vi "v4.vi"() -> ()   [LabVIEW 2015]
uses:
  <vilib>/Utility/miscctls.llb/LVDateTimeRec.ctl
  <vilib>/Analysis/3filter.llb/Filter Passband Type.ctl
  <vilib>/Analysis/8numeric.llb/1D Numeric Integration.vi
  <vilib>/Utility/inputDevices.llb/mouseAcquire.vi
  <vilib>/Utility/cursorutil.llb/Set Cursor (Icon Pict).vi
  <vilib>/Utility/inputDevices.llb/closeMouse.vi
  <vilib>/Utility/cursorutil.llb/Set Cursor (Cursor ID).vi
  <vilib>/Analysis/3filter.llb/Butterworth Filter (DBL).vi
  <vilib>/Utility/file.llb/Write Delimited Spreadsheet (DBL).vi
  <vilib>/Analysis/NI_AALBase.lvlib
  <vilib>/Analysis/NI_AALPro.lvlib
panel:
  out "TM":string
  out "Vertical (cm/px)":dbl
  out "Horizontal (cm/px)":dbl
  out "Alvo_vertical_px":dbl
  out "Alvo_horizontal_px":dbl
  out "Horizontal_atual_px":i32
  out "Vertical_atual_px":i32
  out "cont6":dbl
  out "cont5":dbl
  out "cont4":dbl
  out "cont2":dbl
  out "cont3":dbl
  out "cont1":dbl
  out "codigo":dbl
  out "Area_acel_1_sub":dbl format="%0.4f"
  out "Area_acel_2_sub":dbl format="%0.4f"
  out "Posicao_final_horizontal":dbl
  out "Posicao_final_Vertical":dbl
  out "Posicao_Hori_2_sub":dbl
  out "Posicao_vert_2_sub":dbl
  out "Deslocamento_Horizontal_fill":dbl[](array[numeric])
  out "Deslocamento_Vertical_fill":dbl[](array[numeric])
  out "Deslocamento_tototal_1_sub":dbl[](array[numeric])
  out "Deslocamento_tototal_2_sub":dbl[](array[numeric])
  out "2_sub_mov(s)":dbl
  out "Fim_da_reposta(s)":dbl format="%#.17g"
  out "Inicio_da_reposta(s)":dbl format="%#.17g"
  out "Apresentacao_do_estimulo(s)":dbl format="%#.17g"
  out "Fim_do_warning(s)":dbl format="%#.17g"
  out "Inicio_do_warning(s)":dbl format="%#.17g"
  out "INICIO(s)":dbl format="%#.17g"
  out "Fim_resp_Cluter":T1
  out "Inicio_da_resposta_Cluter":T1
  out "Apresentacao_do_estimulo_Cluter":T1
  out "Fim_do_warning_Cluter":T1
  out "Inicio_do_warning_Cluter":T1
  out "INICIO_Cluter":T1
  out "x/y":dbl
  out "Fim_do_warning":dbl format="%#.10g"
  out "Inicio_do_warning":dbl format="%#.10g"
  out "Posicao_graus_2_sub":dbl
  out "Posicao_cm_2_sub":dbl
  out "ER_no_2_sub":dbl
  out "Posicao_cm_final":dbl
  out "2_sub_mov":dbl format="%#.10g"
  out "Posicao_graus_final":dbl
  out "Graus":dbl[](array[numeric])
  out "n_correcoes":i32
  out "ref_zero_cross":i32[](array[numeric])
  out "Tempo_relativo_pico":dbl
  out "Tempo_para_o_pico":i32
  out "Pico_velocidade":dbl
  out "Fim_resp":dbl format="%#.10g"
  out "Inicio_da_resposta":dbl format="%#.10g"
  out "Vertical_posicao_px":i32[](array[numeric])
  out "Horizontal_posicao_px":i32[](array[numeric])
  out "Jeark":dbl[](array[numeric])
  out "Deslocamento_Horizontal_bruto":dbl[](array[numeric])
  out "Deslocamento_Vertical_bruto":dbl[](array[numeric])
  out "ref_p_inicial_vertical":dbl
  out "posicao_total":dbl[](array[numeric])
  out "INICIO":dbl format="%#.10g"
  out "Apresentacao_do_estimulo":dbl format="%#.10g"
  out "ref_p_inicial_total":dbl
  out "posicao_horizontal":dbl[](array[numeric])
  out "posicao_vertical":dbl[](array[numeric])
  out "Array_x":dbl[](array[numeric])
  out "ref_t_max":dbl
  out "ref_TR":i32
  out "erro radial (cm)":dbl
  out "meta_precisao":dbl
  out "ref_V_alvo":dbl
  out "ref_H_alvo":dbl
  out "ponto_final":dbl
  out "ref_pont":dbl
  out "Deslocamento_Total__bruto":dbl[](array[numeric])
  out "tentativa":i32
  out "referencia de endereco":path
  out "aceleracao":dbl[](array[numeric])
  out "Velocidade":dbl[](array[numeric])
  out "eixo x":dbl[](array[numeric])
  out "Deslocamento_total_filtrado":dbl[](array[numeric])
  out "cursor":picture
  in  "Tab Control":enum32{"Execucao", "Configuração", "Gráficos"}(tab)
  out "tela":picture
  out "ref_p_inicial_horizontal":dbl
  in  "Cor do ponteiro":u32(colorbox)=14421504
  in  "Cor":u32(colorbox)=197379
  in  "Cor":u32(colorbox)
  in  "Tempo do warning estimulo":u32=1000
  in  "Maior":dbl=4000.0
  in  "menor":dbl=2000.0 format="%#_13g"
  in  "Intervalo entre o fim e o inicio da próxima tentativa":u32=4000
  in  "Horizontal (px)":dbl=1366.0
  in  "Horizontal (cm)":dbl=47.2
  in  "Raio":dbl=1.0
  in  "Horizontal":dbl=5.0
  in  "Vertical":dbl=15.0
  in  "Raio":dbl
  in  "Horizontal":dbl
  in  "Vertical":dbl
  in  "Tamanho do ponteiro":dbl=0.2
  in  "Cor":u32(colorbox)
  in  "Raio":dbl
  in  "Horizontal":dbl
  in  "Sincronizar com EEG":bool
  in  "Número de tentativas":i32=10
  in  "Digite aqui o endereço e nome do arquivo":string
  in  "Tempo max  para fechar a tarefa":dbl=1500.0
  in  "Vertical  (cm)":dbl=29.6
  in  "Vertical (px)":dbl=768.0 format="%#_13g"
  in  "Vertical":dbl=20.0 format="%#_13g"
  in  "Horizontal_1":dbl=31.0
  in  "Vertical_1":dbl=15.0
  in  "Raio_1":dbl=0.3
  in  "Horizontal_1":dbl=31.0
  in  "Vertical_1":dbl=15.0 format="%#_13g"
  in  "Cor_1":u32(colorbox)
  in  "Cor_1":u32(colorbox)
  in  "Raio_1":dbl=0.3
  in  "Horizontal_2":dbl
  in  "Vertical_2":dbl
  in  "Raio_2":dbl
  in  "Horizontal_2":dbl
  in  "Vertical_2":dbl=20.0 format="%#_13g"
  in  "Cor_2":u32(colorbox)
  in  "Cor_2":u32(colorbox)
  in  "Raio_2":dbl
  in  "n_tt_1":dbl=10.0
  in  "n_tt_2":dbl
  in  "Horizontal_3":dbl
  in  "Vertical_3":dbl
  in  "Raio_3":dbl
  in  "Horizontal_3":dbl
  in  "Vertical_3":dbl=20.0 format="%#_13g"
  in  "Cor_3":u32(colorbox)
  in  "Cor_3":u32(colorbox)
  in  "Raio_3":dbl
  in  "n_tt_3":dbl
  in  "n_alvos":dbl=1.0
  in  "Horizontal_4":dbl
  in  "Vertical_4":dbl
  in  "Raio_4":dbl
  in  "Horizontal_4":dbl
  in  "Vertical_4":dbl=20.0 format="%#_13g"
  in  "Cor_4":u32(colorbox)
  in  "Cor_4":u32(colorbox)
  in  "Raio_4":dbl
  in  "n_tt_4":dbl
  in  "Raio_5":dbl
  in  "Cor_5":u32(colorbox)
  in  "Cor_5":u32(colorbox)
  in  "Vertical_5":dbl=20.0 format="%#_13g"
  in  "Horizontal_5":dbl
  in  "Raio_5":dbl
  in  "Vertical_5":dbl
  in  "Horizontal_5":dbl
  in  "n_tt_5":dbl
  in  "Raio_6":dbl
  in  "Cor_6":u32(colorbox)
  in  "Cor_6":u32(colorbox)
  in  "Vertical_6":dbl=20.0 format="%#_13g"
  in  "Horizontal_6":dbl
  in  "Raio_6":dbl
  in  "Vertical_6":dbl
  in  "Horizontal_6":dbl
  in  "n_tt_6":dbl
  in  "Tempo max  do tempo de reaçao":dbl=3000.0
  in  "?":path=path "E:/Programas/Apontamento/versao_vertical/cursor_invisivel.cur"
  in  "FB online":bool
  in  "FB terminal":bool=TRUE
  out "Deslocamento":cluster{"X":dbl[], "Y":dbl[]}[](graph) caption="XY Graph"
  out "Velocidade":cluster{"X":dbl[], "Y":dbl[]}[](graph) caption="XY Graph"
  out "Aceleracao":cluster{"X":dbl[], "Y":dbl[]}[](graph) caption="XY Graph"
  out "Jeark":cluster{"X":dbl[], "Y":dbl[]}[](graph) caption="XY Graph"
  out "Tempo de reação":i32
  out "execucao":picture
  out "Tempo de movimento":i32
  out "home":picture
  # "100 h\n500 v"
  # "800 h\n100 v"
  # "Intervalo aleatória entre o prepara e vai"
  # "entre"
  # "Home"
  # "Ponteiro"
  # "Número de alvos"
  # "Digite aqui o endereço do cursor"
  # "Posição do alvo 1 - Preparação"
  # "Posição do alvo 1 - Execução"
  # "Horizontal"
  # "Horizontal"
  # "Raio"
  # "Raio"
  # "Número de tentativas do alvo"
  # "Vertical"
  # "Vertical"
  # "Posição do alvo 2 - Preparação"
  # "Posição do alvo 2 - Execução"
  # "Horizontal"
  # "Horizontal"
  # "Raio"
  # "Raio"
  # "Número de tentativas do alvo"
  # "Vertical"
  # "Desenvolvido por Tércio Apolinário-Souza"
  # "Vertical"
  # "Posição do alvo 3 - Preparação"
  # "Posição do alvo 3 - Execução"
  # "Horizontal"
  # "Horizontal"
  # "Raio"
  # "Raio"
  # "Número de tentativas do alvo"
  # "Vertical"
  # "Vertical"
  # "Posição do alvo 4 - Execução"
  # "Posição do alvo 4 - Preparação"
  # "Horizontal"
  # "Horizontal"
  # "Raio"
  # "Raio"
  # "Número de tentativas do alvo"
  # "Vertical"
  # "Vertical"
  # "Posição do alvo 5 - Preparação"
  # "Posição do alvo 5 - Execução"
  # "Horizontal"
  # "Horizontal"
  # "Raio"
  # "Raio"
  # "Número de tentativas do alvo"
  # "Vertical"
  # "Vertical"
  # "Posição do alvo 6 - Preparação"
  # "Posição do alvo 6 - Execução"
  # "Horizontal"
  # "Horizontal"
  # "Raio"
  # "Raio"
  # "Número de tentativas do alvo"
  # "Vertical"
  # "Vertical"
  # "Linger"
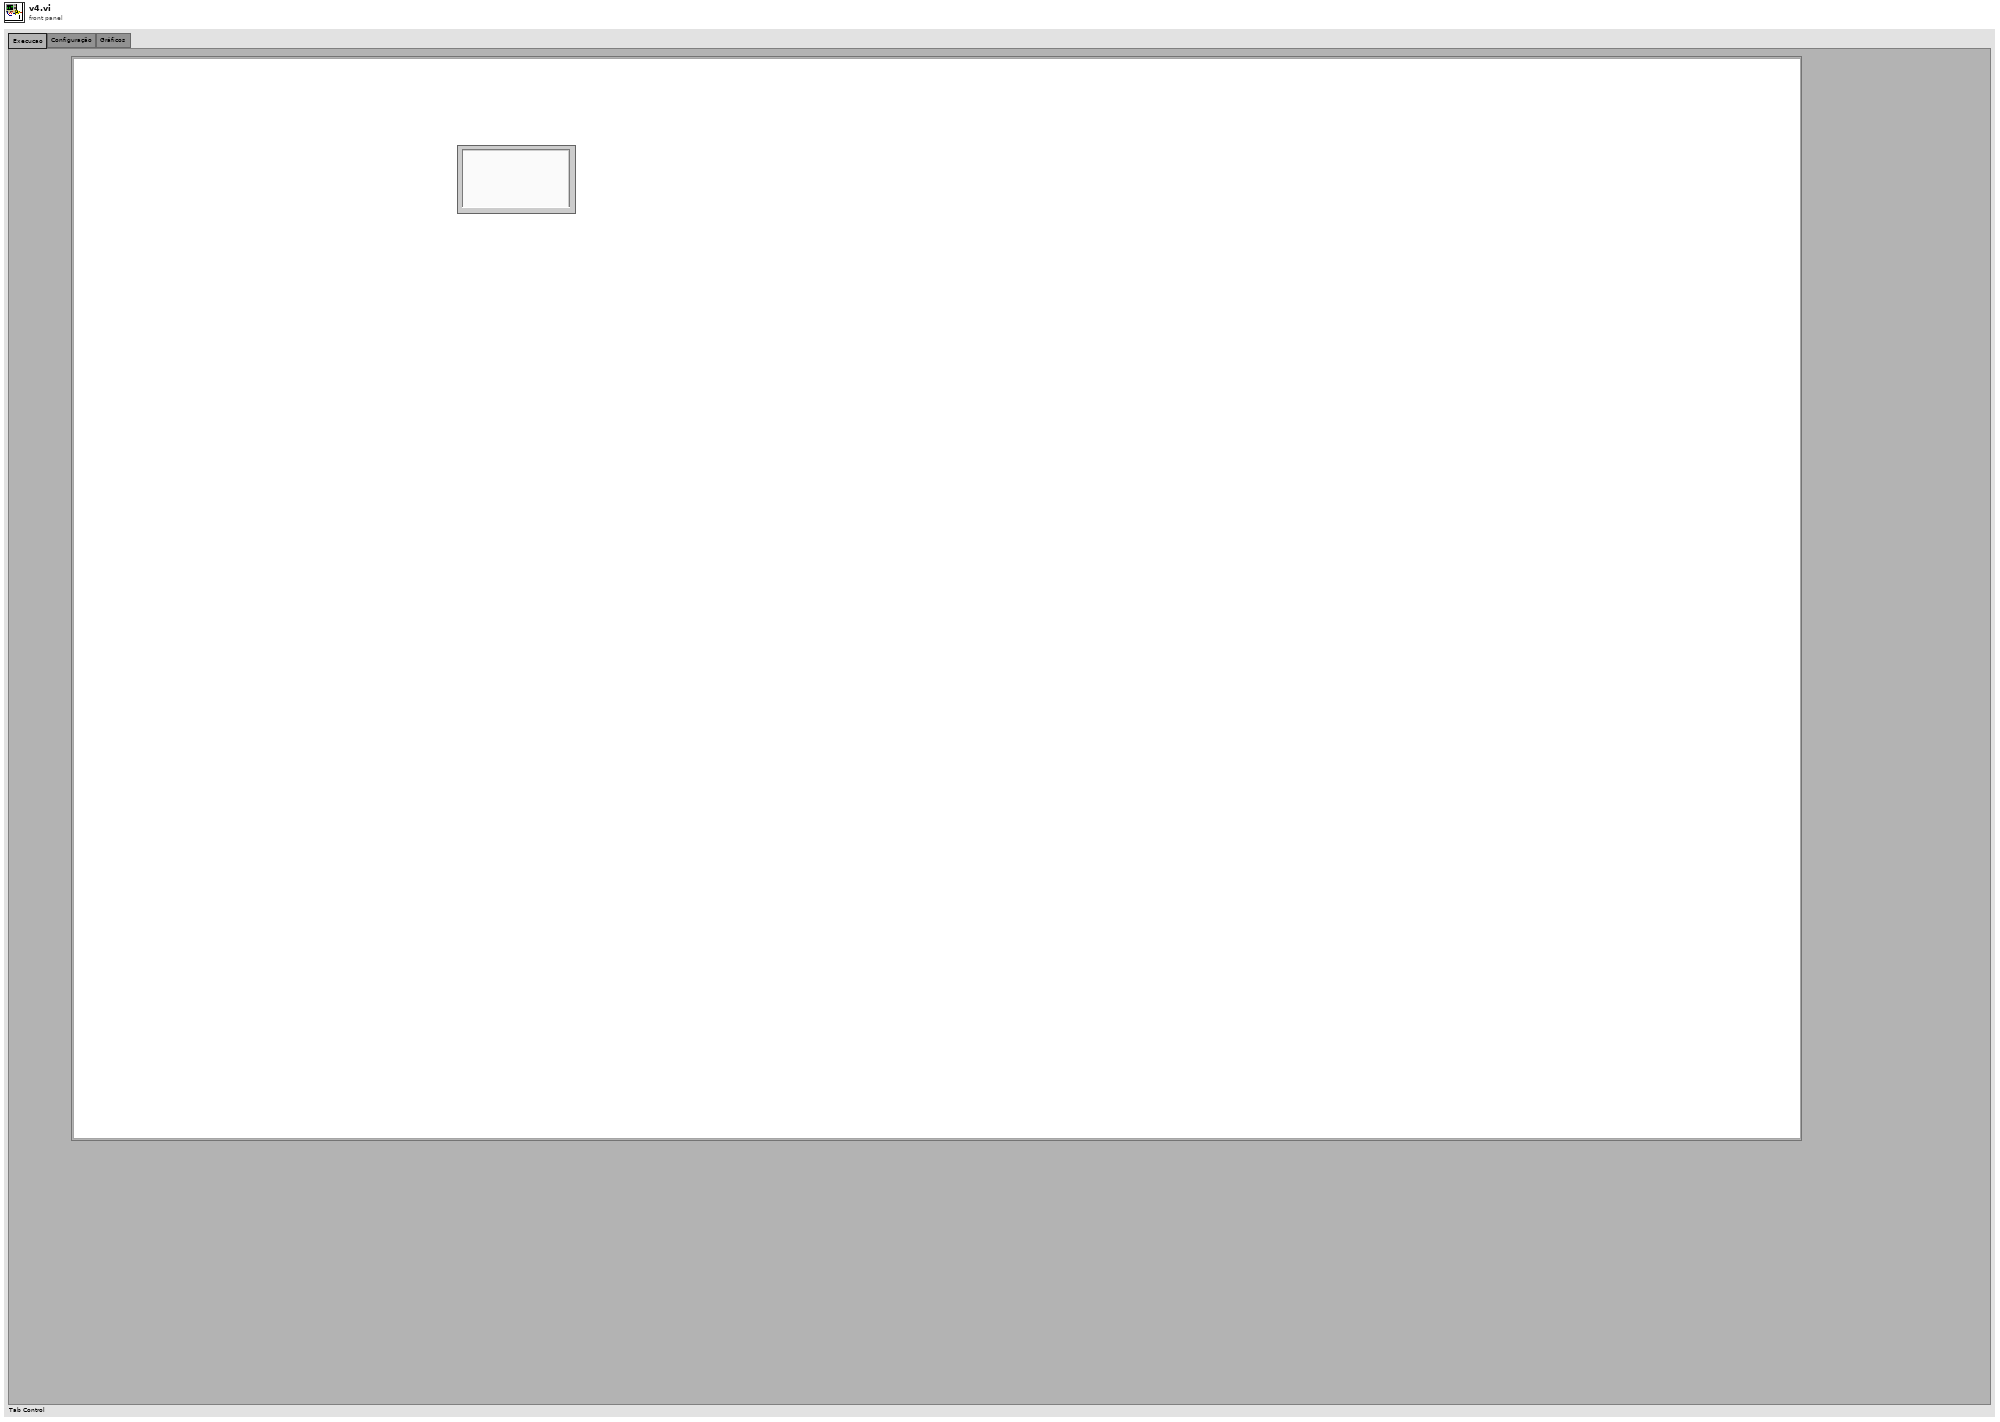
[diagram p1: front panel]
types:
  T1 = typedef "LVDateTimeRec.ctl" = cluster{"fractional second":dbl, "second":i32, "minute":i32, "hour":i32, "day of month":i32, "month":i32, "year":i32, "day of week":i32, "day of year":i32, "DST":i32}
  T2 = typedef "NI_AALBase.lvlib/Filter Passband Type.ctl" = enum32{"Lowpass", "Highpass", "Bandpass", "Bandstop"}
  T3 = cluster{"button 1":bool, "button 2":bool, "button 3":bool, "button 4":bool}
  T4 = cluster{"Horizontal":i32, "Vertical":i32, "Scrolling":i32}
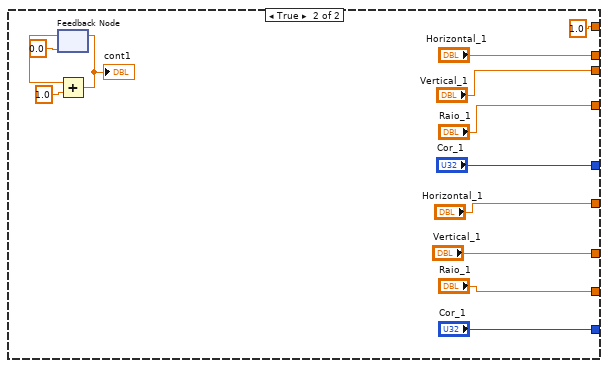
[diagram p4: hidden frame]
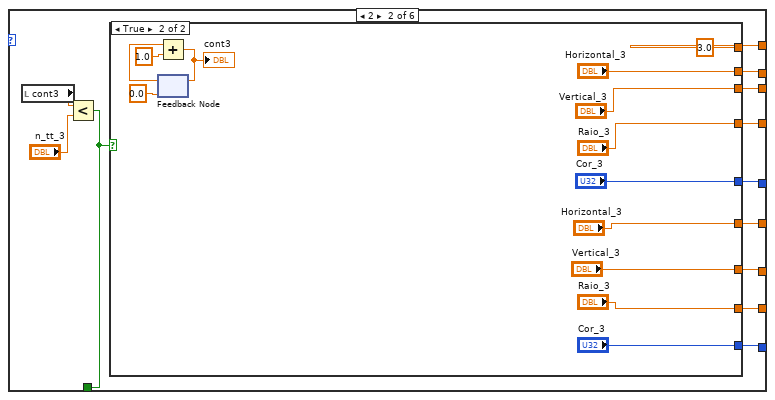
[diagram p5: hidden frame]
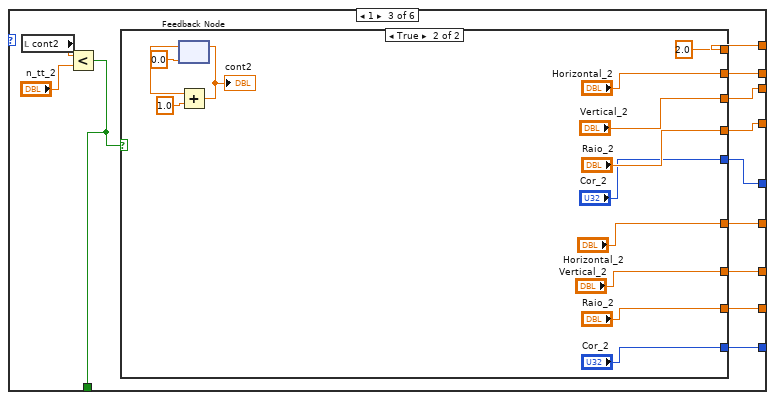
[diagram p7: hidden frame]
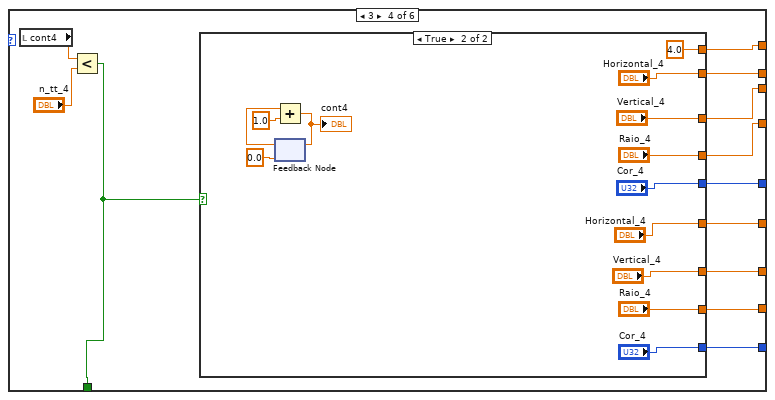
[diagram p9: hidden frame]
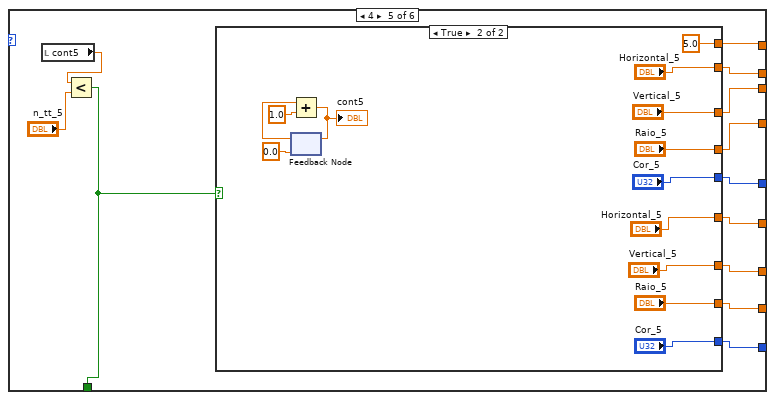
[diagram p11: hidden frame]
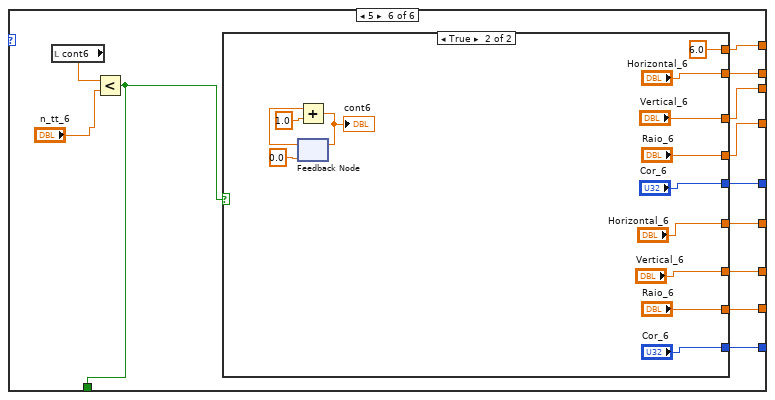
[diagram p13: hidden frame]
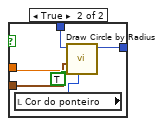
[diagram p20: hidden frame]
diagram:
  w10 = 0.0 ("cont1")
  # "esquerda\ncima\ndireita\nbaixo"
  n1 = local write "cont4"(w10) -> ()
  n2 = local write "cont3"(w10) -> ()
  n3 = local write "cont5"(w10) -> ()
  n4 = local write "cont6"(w10) -> ()
  n5 = local write "cont1"(w10) -> ()
  n6 = local write "cont2"(w10) -> ()
  n7 = for {
    N: "Número de tentativas" -> [_]
    tunnel: [w126] -> w81 mode=indexing
    tunnel: [w125] -> w79 mode=indexing
    tunnel: [w124] -> w77 mode=indexing
    tunnel: [w123] -> w75 mode=indexing
    tunnel: [w122] -> w73 mode=indexing
    tunnel: [w121] -> w71 mode=indexing
    tunnel: [w120] -> w69 mode=indexing
    tunnel: [w119] -> w67 mode=indexing
    tunnel: [w118] -> w65 mode=indexing
    tunnel: [w117] -> w63 mode=indexing
    tunnel: [w116] -> w61 mode=indexing
    tunnel: [w115] -> w59 mode=indexing
    tunnel: [w114] -> w57 mode=indexing
    tunnel: [w113] -> w55 mode=indexing
    tunnel: [w112] -> w52 mode=indexing
    tunnel: [w111] -> w51 mode=indexing
    tunnel: [w110] -> w48 mode=indexing
    tunnel: [w109] -> w47 mode=indexing
    tunnel: [w108] -> w45 mode=indexing
    tunnel: [w107] -> w43 mode=indexing
    tunnel: [w106] -> w41 mode=indexing
    tunnel: [w105] -> w39 mode=indexing
    tunnel: [w104] -> w37 mode=indexing
    tunnel: [w103] -> w35 mode=indexing
    tunnel: [w102] -> w32 mode=indexing
    tunnel: [w101] -> w30 mode=indexing
    tunnel: [w100] -> w29 mode=indexing
    tunnel: [w99] -> w27 mode=indexing
    tunnel: [w98] -> w26 mode=indexing
    tunnel: [w97] -> w24 mode=indexing
    tunnel: [w96] -> w22 mode=indexing
    tunnel: [w95] -> w13 mode=indexing
    tunnel: [w94] -> w19 mode=indexing
    tunnel: [w93] -> w17 mode=indexing
    tunnel: [w92] -> w16 mode=indexing
    tunnel: [w91] -> w9 mode=indexing
    tunnel: [w90] -> w8 mode=indexing
    tunnel: [w89] -> w6 mode=indexing
    tunnel: [w88] -> w4 mode=indexing
    tunnel: [w87] -> w2 mode=indexing
    i -> [w141]
    n8 = Increment(x=w141) -> (x+1=→"tentativa":i32)
    n9 = flat-sequence {
      tunnel: w141 -> [w143]
      tunnel: [w510] -> w139
      tunnel: [w509] -> w134
      tunnel: w139 -> [w608]
      tunnel: [w603] -> w136
      tunnel: [w602] -> w135
      tunnel: w134 -> [w611]
      tunnel: [w601] -> w133
      tunnel: [w696] -> w138
      tunnel: w136 -> [w685]
      tunnel: w135 -> [w679]
      tunnel: w133 -> [w678]
      tunnel: [w676] -> w132
      tunnel: [w677] -> w130
      tunnel: w138 -> [w715]
      tunnel: [w715] -> w137
      tunnel: w132 -> [w702]
      tunnel: [w702] -> w131
      tunnel: w130 -> [w700]
      tunnel: [w700] -> w129
      tunnel: w137 -> [w747]
      tunnel: w131 -> [w744]
      tunnel: w129 -> [w741]
      tunnel: [w880] -> w128
      tunnel: [w880] -> w127
      tunnel: w128 -> [w916]
      tunnel: w127 -> [w928]
      tunnel: [w1125] -> w126
      tunnel: [w1124] -> w125
      tunnel: [w1123] -> w124
      tunnel: [w1122] -> w123
      tunnel: [w1121] -> w122
      tunnel: [w1120] -> w121
      tunnel: [w1119] -> w120
      tunnel: [w1118] -> w119
      tunnel: [w1117] -> w118
      tunnel: [w1116] -> w117
      tunnel: [w1115] -> w116
      tunnel: [w1114] -> w115
      tunnel: [w1113] -> w114
      tunnel: [w1112] -> w113
      tunnel: [w1111] -> w112
      tunnel: [w1110] -> w111
      tunnel: [w1109] -> w110
      tunnel: [w1108] -> w109
      tunnel: [w1107] -> w108
      tunnel: [w1106] -> w107
      tunnel: [w1105] -> w106
      tunnel: [w1104] -> w105
      tunnel: [w1103] -> w104
      tunnel: [w1102] -> w103
      tunnel: [w1101] -> w102
      tunnel: [w1100] -> w101
      tunnel: [w1099] -> w100
      tunnel: [w1098] -> w99
      tunnel: [w1097] -> w98
      tunnel: [w1096] -> w97
      tunnel: [w1095] -> w96
      tunnel: [w1085] -> w95
      tunnel: [w1082] -> w94
      tunnel: [w1094] -> w93
      tunnel: [w1093] -> w92
      tunnel: [w1081] -> w91
      tunnel: [w1080] -> w90
      tunnel: [w1079] -> w89
      tunnel: [w1078] -> w88
      tunnel: [w1077] -> w87
      frame #0 {
        n10 = Equal?(x=w143, y=0) -> (x = y?=w147:bool)
        n11 = And(x="Sincronizar com EEG", y=w147) -> (x .and. y?=w145:bool)
        n12 = case shown="True" w145 {
          frame False {
          }
          frame True {
            n13 = call <vilib>:"Initialize Mouse.vi"() -> ("error out"=w149:errorcluster, "device ID"=w150:refnum<k1>)  [unwired: 10 in]
            n14 = while {
              tunnel: w150 -> [w156]
              tunnel: w149 -> [w155]
              tunnel: enum16{"RELATIVE", "ABSOLUTE"}."ABSOLUTE" ("key mode") -> [w154]
              stop <- w152 stop-if-true
              n15 = call-poly <vilib>:"Acquire Input Data.vi"("device ID"=w156, "key mode"=w154, "error in (no error)"=w155) -> ("button info"=w153:T3)  [unwired: 13 in, 3 out]
              n16 = Unbundle(w153) -> ("button 1"=w151:bool)  [unwired: 3 out]
              n17 = case shown="True" w151 {
                tunnel: [_ TRUE] -> w152
                frame False {
                }
                frame True {
                  n18 = Get Date/Time In Seconds() -> (seconds since 1Jan1904=w158:timestamp)
                  n19 = Format Date/Time String(time format string (%c)="%H%M%S%4u", seconds (now)=w158) -> (date/time string=w160:string)  [unwired: 1 in]
                  n20 = Fract/Exp String To Number(use system decimal point (T)=TRUE, string=w160) -> (number=→"INICIO":dbl)  [unwired: 2 in, 1 out]
                  n21 = Seconds To Date/Time(time stamp (now)=w158) -> (date time rec=→"INICIO_Cluter":T1)  [unwired: 1 in]
                }
              }
            }
          }
        }
        n22 = property on="TM" class="Str"("Visible"=FALSE) -> ()  [unwired: 2 in, 2 out]
      }
      frame #1 {
        n23 = Divide(x="Vertical  (cm)", y="Vertical (px)") -> (x/y=→"Vertical (cm/px)":dbl)
        n24 = Divide(x="Horizontal (cm)", y="Horizontal (px)") -> (x/y=→"Horizontal (cm/px)":dbl)
      }
      frame #2 {
        # "execucao"
        # "Preparacao"
        # "Selecioar alvo"
        n25 = while {
          tunnel: [w188] -> w178
          tunnel: [w187] -> w177
          tunnel: [w186] -> w176
          tunnel: [w185] -> w175
          tunnel: [w184] -> w171
          tunnel: [w183] -> w170
          tunnel: [w182] -> w174
          tunnel: [w181] -> w173
          tunnel: [w179] -> w172
          stop <- w194 stop-if-true
          n26 = Random Number (0-1)() -> (number: 0 to 1=w192:dbl)
          n27 = Multiply(x=w192, y=100.0) -> (x*y=w191:dbl)
          n28 = To Byte Integer(number=w191) -> (8bit integer=w190:i8)
          n29 = Quotient & Remainder(x=w190, y="n_alvos") -> (x-y*floor(x/y)=w189:dbl)  [unwired: 1 out]
          n30 = case shown="0, Default" w189 {
            tunnel: [w206 w231 w256 w278 w306 w327] -> w179
            tunnel: [w204 w229 w254 w280 w296 w329] -> w194
            tunnel: [w203 w228 w253 w277 w305 w328] -> w188
            tunnel: [w202 w227 w252 w276 w304 w326] -> w187
            tunnel: [w201 w226 w251 w275 w303 w325] -> w186
            tunnel: [w200 w225 w250 w274 w302 w324] -> w185
            tunnel: [w199 w224 w249 w273 w301 w323] -> w184
            tunnel: [w198 w223 w248 w272 w300 w322] -> w183
            tunnel: [w197 w222 w247 w271 w299 w321] -> w182
            tunnel: [w196 w221 w246 w270 w298 w320] -> w181
            frame 0, Default {
              n31 = local read "cont1"() -> (w205:dbl)
              n32 = Less?(x=w205, y="n_tt_1") -> (x < y?=w204:bool)
              n33 = case shown="False" w204 {
                tunnel: [_ 1.0] -> w206
                tunnel: [_ "Horizontal_1"] -> w203
                tunnel: [_ "Vertical_1"] -> w202
                tunnel: [_ "Raio_1"] -> w201
                tunnel: [_ "Cor_1"] -> w200
                tunnel: [_ "Horizontal_1"] -> w199
                tunnel: [_ "Vertical_1"] -> w198
                tunnel: [_ "Raio_1"] -> w197
                tunnel: [_ "Cor_1"] -> w196
                frame False {
                }
                frame True {
                  n34 = feedback #1(0.0) -> (w218:dbl)
                  n35 = Add(x=w218, y=1.0) -> (x+y=w215:dbl)
                  "cont1" <- w215
                  n36 = feedback-in #1(w215) -> ()
                }
              }
            }
            frame 2 {
              n37 = local read "cont3"() -> (w230:dbl)
              n38 = Less?(x=w230, y="n_tt_3") -> (x < y?=w229:bool)
              n39 = case shown="True" w229 {
                tunnel: [_ 3.0] -> w231
                tunnel: [_ "Horizontal_3"] -> w228
                tunnel: [_ "Vertical_3"] -> w227
                tunnel: [_ "Raio_3"] -> w226
                tunnel: [_ "Cor_3"] -> w225
                tunnel: [_ "Horizontal_3"] -> w224
                tunnel: [_ "Vertical_3"] -> w223
                tunnel: [_ "Raio_3"] -> w222
                tunnel: [_ "Cor_3"] -> w221
                frame False {
                }
                frame True {
                  n40 = feedback #2(0.0) -> (w242:dbl)
                  n41 = Add(x=w242, y=1.0) -> (x+y=w243:dbl)
                  "cont3" <- w243
                  n42 = feedback-in #2(w243) -> ()
                }
              }
            }
            frame 1 {
              n43 = local read "cont2"() -> (w255:dbl)
              n44 = Less?(x=w255, y="n_tt_2") -> (x < y?=w254:bool)
              n45 = case shown="True" w254 {
                tunnel: [_ 2.0] -> w256
                tunnel: [_ "Horizontal_2"] -> w253
                tunnel: [_ "Vertical_2"] -> w252
                tunnel: [_ "Raio_2"] -> w251
                tunnel: [_ "Cor_2"] -> w250
                tunnel: [_ "Horizontal_2"] -> w249
                tunnel: [_ "Vertical_2"] -> w248
                tunnel: [_ "Raio_2"] -> w247
                tunnel: [_ "Cor_2"] -> w246
                frame False {
                }
                frame True {
                  n46 = feedback #3(0.0) -> (w267:dbl)
                  n47 = Add(x=w267, y=1.0) -> (x+y=w268:dbl)
                  "cont2" <- w268
                  n48 = feedback-in #3(w268) -> ()
                }
              }
            }
            frame 3 {
              n49 = local read "cont4"() -> (w279:dbl)
              n50 = Less?(x=w279, y="n_tt_4") -> (x < y?=w280:bool)
              n51 = case shown="True" w280 {
                tunnel: [_ 4.0] -> w278
                tunnel: [_ "Horizontal_4"] -> w277
                tunnel: [_ "Vertical_4"] -> w276
                tunnel: [_ "Raio_4"] -> w275
                tunnel: [_ "Cor_4"] -> w274
                tunnel: [_ "Horizontal_4"] -> w273
                tunnel: [_ "Vertical_4"] -> w272
                tunnel: [_ "Raio_4"] -> w271
                tunnel: [_ "Cor_4"] -> w270
                frame False {
                }
                frame True {
                  n52 = feedback #4(0.0) -> (w293:dbl)
                  n53 = Add(x=w293, y=1.0) -> (x+y=w294:dbl)
                  "cont4" <- w294
                  n54 = feedback-in #4(w294) -> ()
                }
              }
            }
            frame 4 {
              n55 = local read "cont5"() -> (w295:dbl)
              n56 = Less?(x=w295, y="n_tt_5") -> (x < y?=w296:bool)
              n57 = case shown="True" w296 {
                tunnel: [_ 5.0] -> w306
                tunnel: [_ "Horizontal_5"] -> w305
                tunnel: [_ "Vertical_5"] -> w304
                tunnel: [_ "Raio_5"] -> w303
                tunnel: [_ "Cor_5"] -> w302
                tunnel: [_ "Horizontal_5"] -> w301
                tunnel: [_ "Vertical_5"] -> w300
                tunnel: [_ "Raio_5"] -> w299
                tunnel: [_ "Cor_5"] -> w298
                frame False {
                }
                frame True {
                  n58 = feedback #5(0.0) -> (w318:dbl)
                  n59 = Add(x=w318, y=1.0) -> (x+y=w319:dbl)
                  "cont5" <- w319
                  n60 = feedback-in #5(w319) -> ()
                }
              }
            }
            frame 5 {
              n61 = local read "cont6"() -> (w330:dbl)
              n62 = Less?(x=w330, y="n_tt_6") -> (x < y?=w329:bool)
              n63 = case shown="True" w329 {
                tunnel: [_ 6.0] -> w327
                tunnel: [_ "Horizontal_6"] -> w328
                tunnel: [_ "Vertical_6"] -> w326
                tunnel: [_ "Raio_6"] -> w325
                tunnel: [_ "Cor_6"] -> w324
                tunnel: [_ "Horizontal_6"] -> w323
                tunnel: [_ "Vertical_6"] -> w322
                tunnel: [_ "Raio_6"] -> w321
                tunnel: [_ "Cor_6"] -> w320
                frame False {
                }
                frame True {
                  n64 = feedback #6(0.0) -> (w343:dbl)
                  n65 = Add(x=w343, y=1.0) -> (x+y=w344:dbl)
                  "cont6" <- w344
                  n66 = feedback-in #6(w344) -> ()
                }
              }
            }
          }
        }
        "codigo" <- w172
        n67 = local write "Horizontal"(w178) -> ()
        n68 = local write "Vertical"(w177) -> ()
        n69 = local write "Horizontal"(w171) -> ()
        n70 = local write "Raio"(w174) -> ()
        n71 = local write "Cor"(w175) -> ()
        n72 = local write "Vertical"(w170) -> ()
        n73 = local write "Raio"(w176) -> ()
        n74 = local write "Cor"(w173) -> ()
      }
      frame #3 {
        # "voltar o mouse ao normal"
        # "Preparação"
        n75 = call <vilib>:"Initialize Mouse.vi"() -> ("error out"=w348:errorcluster, "device ID"=w349:refnum<k1>)  [unwired: 10 in]
        n76 = while {
          tunnel: w349 -> [w401]
          tunnel: w348 -> [w394]
          tunnel: [w376] -> w347
          tunnel: [w395] -> w346
          stop <- w396 stop-if-true
          # "Alvo 1"
          n77 = local read "Vertical  (cm)"() -> (w374:dbl)
          n78 = local read "Horizontal (cm/px)"() -> (w353:dbl)
          n79 = call-poly <vilib>:"Acquire Input Data.vi"("device ID"=w401, "error in (no error)"=w394) -> ("device ID"=w376:refnum<k1>, "axis info"=w400:T4, "error out"=w395:errorcluster)  [unwired: 14 in, 1 out]
          n80 = Subtract(x=w374, y="Vertical") -> (x-y=w373:dbl)
          n81 = Divide(x=w373, y=w353) -> (x/y=w352:dbl)
          n82 = Unbundle By Name(w400) -> ("Vertical"=w368:i32, "Horizontal"=w371:i32)
          n83 = Divide(x="Horizontal", y=w353) -> (x/y=w377:dbl)
          n84 = Divide(x="Raio", y=w353) -> (x/y=w360:dbl)
          "x/y" <- w360
          n85 = Bundle(w377, w352) -> (w384:cluster{dbl, dbl})  [unwired: 1 in]
          n86 = Quotient & Remainder(x=w377, y=1.0) -> (floor(x/y)=w370:dbl)  [unwired: 1 out]
          n87 = Quotient & Remainder(x=w352, y=1.0) -> (floor(x/y)=w367:dbl)  [unwired: 1 out]
          n88 = call <vilib>:"Draw Circle by Radius.vi"("color(black)"="Cor", "fill?(F)"=TRUE, "pixel center"=w384, "radius"=w360) -> ("new picture"=w385:picture)  [unwired: 7 in]
          "home" <- w385
          n89 = Subtract(x=w371, y=w370) -> (x-y=w369:dbl)
          n90 = local read "Horizontal (cm/px)"() -> (w386:dbl)
          n91 = Subtract(x=w368, y=w367) -> (x-y=w366:dbl)
          n92 = Absolute Value(x=w369) -> (abs(x)=w363:dbl)
          n93 = local read "Vertical  (cm)"() -> (w375:dbl)
          n94 = local read "Vertical"() -> (w356:dbl)
          n95 = local read "Horizontal (cm/px)"() -> (w381:dbl)
          n96 = local read "Raio"() -> (w357:dbl)
          n97 = local read "Horizontal"() -> (w358:dbl)
          n98 = Absolute Value(x=w366) -> (abs(x)=w362:dbl)
          n99 = Divide(x=w360, y=2.0) -> (x/y=w359:dbl)
          n100 = Less Or Equal?(x=w362, y=w359) -> (x <= y?=w364:bool)
          n101 = Less Or Equal?(x=w363, y=w359) -> (x <= y?=w365:bool)
          n102 = Bundle("Horizontal"=w371, "Vertical"=w368) -> (w399:cluster{"Horizontal":i32, "Vertical":i32})  [unwired: 1 in]
          n103 = Subtract(x=w375, y=w356) -> (x-y=w372:dbl)
          n104 = And(x=w364, y=w365) -> (x .and. y?=w396:bool)
          n105 = Divide(x=w372, y=w386) -> (x/y=w350:dbl)
          "ref_V_alvo" <- w350
          n106 = Divide(x=w357, y=w386) -> (x/y=w390:dbl)
          n107 = Divide(x=w358, y=w386) -> (x/y=w351:dbl)
          "ref_H_alvo" <- w351
          n108 = Divide(x="Tamanho do ponteiro", y=w381) -> (x/y=w380:dbl)
          "ref_pont" <- w380
          n109 = Bundle(w351, w350) -> (w387:cluster{dbl, dbl})  [unwired: 1 in]
          n110 = local read "Cor"() -> (w355:u32)
          n111 = call <vilib>:"Draw Circle by Radius.vi"("color(black)"=w355, "fill?(F)"=TRUE, "pixel center"=w387, "radius"=w390, "picture"=w385) -> ("new picture"=w389:picture)  [unwired: 6 in]
          "cursor" <- w389
          n112 = call <vilib>:"Draw Circle by Radius.vi"("color(black)"="Cor do ponteiro", "fill?(F)"=TRUE, "pixel center"=w399, "radius"=w380, "picture"=w389) -> ("new picture"=→"tela":picture)  [unwired: 6 in]
        }
        n113 = call-poly <vilib>:"Set Cursor.vi"("icon"=i16 0 ("cursor resource ID")) -> ()  [unwired: 9 in, 2 out]
        n114 = call-poly <vilib>:"Close Input Device.vi"("error in (no error)"=w346, "device ID"=w347) -> ()  [unwired: 8 in, 1 out]
      }
      frame #4 {
      }
      frame #5 {
        n115 = case shown="True" TRUE {
          frame False {
          }
          frame True {
            n116 = Get Date/Time In Seconds() -> (seconds since 1Jan1904=w409:timestamp)
            n117 = Format Date/Time String(time format string (%c)="%H%M%S%4u", seconds (now)=w409) -> (date/time string=w411:string)  [unwired: 1 in]
            n118 = Fract/Exp String To Number(use system decimal point (T)=TRUE, string=w411) -> (number=→"Inicio_do_warning":dbl)  [unwired: 2 in, 1 out]
            n119 = Seconds To Date/Time(time stamp (now)=w409) -> (date time rec=→"Inicio_do_warning_Cluter":T1)  [unwired: 1 in]
          }
        }
        n120 = Wait (ms)(milliseconds to wait="Tempo do warning estimulo") -> ()  [unwired: 1 out]
        n121 = call <vilib>:"Beep.vi"("use system alert? (T)"=FALSE, "duration (msec)"=u32 200, "frequency (Hz)"=u32 500) -> ()  [unwired: 9 in]
      }
      frame #6 {
        # "ocultar o mouse"
        # "intervalo entre 1 a 3 segundo"
        # "Isso serve para apagar"
        n122 = case shown="True" TRUE {
          frame False {
          }
          frame True {
            n123 = Get Date/Time In Seconds() -> (seconds since 1Jan1904=w425:timestamp)
            n124 = Format Date/Time String(time format string (%c)="%H%M%S%4u", seconds (now)=w425) -> (date/time string=w428:string)  [unwired: 1 in]
            n125 = Fract/Exp String To Number(use system decimal point (T)=TRUE, string=w428) -> (number=→"Fim_do_warning":dbl)  [unwired: 2 in, 1 out]
            n126 = Seconds To Date/Time(time stamp (now)=w425) -> (date time rec=→"Fim_do_warning_Cluter":T1)  [unwired: 1 in]
          }
        }
        n127 = Random Number (0-1)() -> (number: 0 to 1=w418:dbl)
        n128 = Subtract(x="Maior", y=1.0) -> (x-y=w423:dbl)
        n129 = call <vilib>:"Draw Circle by Radius.vi"() -> ("new picture"=w417:picture)  [unwired: 11 in]
        n130 = Multiply(x=w423, y=w418) -> (x*y=w419:dbl)
        n131 = Add(x=w419, y="menor") -> (x+y=w424:dbl)
        n132 = local write "tela"(w417) -> ()
        n133 = Wait (ms)(milliseconds to wait=w424) -> ()  [unwired: 1 out]
        n134 = call <vilib>:"Create Cursor From File.vi"("cursor file"="?") -> ("cursor ID"=w415:refnum<k1>)  [unwired: 9 in, 1 out]
        n135 = call-poly <vilib>:"Set Cursor.vi"("cursor ID"=w415) -> ()  [unwired: 9 in, 2 out]
      }
      frame #7 {
        w439 = dbl[] [0.0]
        # "Tempo reação"
        n136 = call <vilib>:"Initialize Mouse.vi"() -> ("error out"=w441:errorcluster, "device ID"=w442:refnum<k1>)  [unwired: 10 in]
        n137 = case shown="True" TRUE {
          frame False {
          }
          frame True {
            n138 = Get Date/Time In Seconds() -> (seconds since 1Jan1904=w443:timestamp)
            n139 = Format Date/Time String(time format string (%c)="%H%M%S%4u", seconds (now)=w443) -> (date/time string=w446:string)  [unwired: 1 in]
            n140 = Fract/Exp String To Number(use system decimal point (T)=TRUE, string=w446) -> (number=→"Apresentacao_do_estimulo":dbl)  [unwired: 2 in, 1 out]
            n141 = Seconds To Date/Time(time stamp (now)=w443) -> (date time rec=→"Apresentacao_do_estimulo_Cluter":T1)  [unwired: 1 in]
          }
        }
        n142 = while {
          tunnel: w442 -> [w498]
          tunnel: w441 -> [w497]
          tunnel: [w494] -> w435
          tunnel: [w496] -> w440
          shift-right: [w493] -> _
          shift-left: w439 -> [w492]
          shift-left: w439 -> [w489]
          tunnel: [w454] -> w437
          i -> [w454]
          stop <- w455 stop-if-true
          n143 = local read "Horizontal (cm/px)"() -> (w477:dbl)
          n144 = local read "Horizontal"() -> (w461:dbl)
          n145 = local read "Vertical  (cm)"() -> (w463:dbl)
          n146 = local read "Vertical"() -> (w460:dbl)
          n147 = Divide(x="Tempo max  do tempo de reaçao", y=10.0) -> (x/y=w451:dbl)
          n148 = call-poly <vilib>:"Acquire Input Data.vi"("device ID"=w498, "error in (no error)"=w497) -> ("device ID"=w494:refnum<k1>, "axis info"=w467:T4, "error out"=w496:errorcluster)  [unwired: 14 in, 1 out]
          n149 = Subtract(x=w454, y=2) -> (x-y=w490:i32)
          n150 = Subtract(x=w463, y=w460) -> (x-y=w462:dbl)
          n151 = local read "Raio"() -> (w458:dbl)
          n152 = Divide(x=w462, y=w477) -> (x/y=w449:dbl)
          "Alvo_vertical_px" <- w449
          n153 = Divide(x=w461, y=w477) -> (x/y=w450:dbl)
          "Alvo_horizontal_px" <- w450
          n154 = Unbundle By Name(w467) -> ("Vertical"=w470:i32, "Horizontal"=w471:i32)
          n155 = Wait Until Next ms Multiple(millisecond multiple=u32 10) -> ()  [unwired: 1 out]
          n156 = Index Array(array=w489, index=w490) -> (element=w486:dbl)
          n157 = Index Array(array=w492, index=w454) -> (element=w487:dbl)
          n158 = local read "home"() -> (w476:picture)
          n159 = Bundle(w450, w449) -> (w479:cluster{dbl, dbl})  [unwired: 1 in]
          n160 = Divide(x=w458, y=w477) -> (x/y=w478:dbl)
          n161 = Subtract(x=w487, y=w486) -> (x-y=w485:dbl)
          n162 = local read "Cor"() -> (w459:u32)
          n163 = feedback #7(0.0) -> (w484:dbl)
          n164 = Not Equal To 0?(x=w485) -> (x != 0?=w481:bool)
          n165 = Square(x=w470) -> (x^2=w495:i32)
          n166 = Square(x=w471) -> (x^2=w466:i32)
          n167 = case shown="True" w481 {
            tunnel: [_ w500] -> w483
            tunnel: w484 -> [_ w502]
            tunnel: [_ w501] -> w456
            frame False {
            }
            frame True {
              n168 = Increment(x=w502) -> (x+1=w500:dbl)
              n169 = Greater Or Equal?(x=w500, y=3.0) -> (x >= y?=w501:bool)
            }
          }
          n170 = feedback-in #7(w483) -> ()
          n171 = call <vilib>:"Draw Circle by Radius.vi"("color(black)"=w459, "fill?(F)"=TRUE, "pixel center"=w479, "radius"=w478, "picture"=w476) -> ("new picture"=w475:picture)  [unwired: 6 in]
          "execucao" <- w475
          n172 = Add(x=w495, y=w466) -> (x+y=w465:i32)
          n173 = local read "ref_pont"() -> (w473:dbl)
          n174 = Square Root(x=w465) -> (sqrt(x)=w464:dbl)
          n175 = Bundle("Horizontal"=w471, "Vertical"=w470) -> (w472:cluster{"Horizontal":i32, "Vertical":i32})  [unwired: 1 in]
          n176 = Greater?(x=w454, y=w451) -> (0:w457:bool)
          n177 = Or(x=w456, y=w457) -> (x .or. y?=w455:bool)
          n178 = Insert Into Array(array=w492, new element=w464) -> (w493:dbl[])  [unwired: 1 in]
          n179 = local read "Cor do ponteiro"() -> (w468:u32)
          n180 = call <vilib>:"Draw Circle by Radius.vi"("color(black)"=w468, "fill?(F)"=TRUE, "pixel center"=w472, "radius"=w473, "picture"=w475) -> ("new picture"=w474:picture)  [unwired: 6 in]
          n181 = local write "tela"(w474) -> ()
          "ref_TR" <- w454
        }
        n182 = call <vilib>:"Beep.vi"("use system alert? (T)"=FALSE, "duration (msec)"=u32 200, "frequency (Hz)"=u32 700) -> ()  [unwired: 9 in]
        n183 = Multiply(x=w437, y=10) -> (x*y=→"Tempo de reação":i32)
        n184 = call-poly <vilib>:"Close Input Device.vi"("error in (no error)"=w440, "device ID"=w435) -> ()  [unwired: 8 in, 1 out]
      }
      frame #8 {
        n185 = local read "ref_TR"() -> (w506:i32)
        n186 = Divide(x="Tempo max  para fechar a tarefa", y=10.0) -> (x/y=w505:dbl)
        n187 = Subtract(x=w505, y=w506) -> (x-y=w507:dbl)
        n188 = Absolute Value(x=w507) -> (abs(x)=→"ref_t_max":dbl)
      }
      frame #9 {
        w512 = i32[] [0]
        w521 = dbl[] [0.0]
        # "Execução"
        n189 = case shown="True" TRUE {
          frame False {
          }
          frame True {
            n190 = Get Date/Time In Seconds() -> (seconds since 1Jan1904=w524:timestamp)
            n191 = Format Date/Time String(time format string (%c)="%H%M%S%4u", seconds (now)=w524) -> (date/time string=w527:string)  [unwired: 1 in]
            n192 = Fract/Exp String To Number(use system decimal point (T)=TRUE, string=w527) -> (number=→"Inicio_da_resposta":dbl)  [unwired: 2 in, 1 out]
            n193 = Seconds To Date/Time(time stamp (now)=w524) -> (date time rec=→"Inicio_da_resposta_Cluter":T1)  [unwired: 1 in]
          }
        }
        n194 = call <vilib>:"Initialize Mouse.vi"() -> ("error out"=w517:errorcluster, "device ID"=w518:refnum<k1>)  [unwired: 10 in]
        n195 = while {
          tunnel: w518 -> [w571]
          tunnel: w517 -> [w575]
          tunnel: [w574] -> w523
          tunnel: [w572] -> w522
          shift-right: [w549] -> _
          shift-left: w521 -> [w556]
          shift-left: w521 -> [w566]
          tunnel: [w544] -> w516
          shift-right: [w551] -> w513
          shift-left: w521 -> [w550]
          shift-right: [w542] -> w509
          shift-left: w512 -> [w541]
          shift-right: [w538] -> w510
          shift-left: w512 -> [w537]
          i -> [w544]
          stop <- w545 stop-if-true
          n196 = call-poly <vilib>:"Acquire Input Data.vi"("device ID"=w571, "error in (no error)"=w575) -> ("device ID"=w572:refnum<k1>, "axis info"=w573:T4, "error out"=w574:errorcluster)  [unwired: 14 in, 1 out]
          n197 = Subtract(x=w544, y=2) -> (x-y=w568:i32)
          n198 = Wait Until Next ms Multiple(millisecond multiple=u32 10) -> ()  [unwired: 1 out]
          n199 = Index Array(array=w566, index=w568) -> (element=w565:dbl)
          n200 = Index Array(array=w556, index=w544) -> (element=w554:dbl)
          n201 = Unbundle By Name(w573) -> ("Vertical"=w540:i32, "Horizontal"=w531:i32)
          "Vertical_atual_px" <- w540
          "Horizontal_atual_px" <- w531
          n202 = local read "ref_pont"() -> (w532:dbl)
          n203 = Subtract(x=w554, y=w565) -> (x-y=w555:dbl)
          n204 = feedback #8(0.0) -> (w563:dbl)
          n205 = Equal To 0?(x=w555) -> (x = 0?=w561:bool)
          n206 = local read "execucao"() -> (w533:picture)
          n207 = local read "FB online"() -> (w530:bool)
          n208 = Square(x=w540) -> (x^2=w570:i32)
          n209 = Square(x=w531) -> (x^2=w569:i32)
          n210 = case shown="True" w561 {
            tunnel: [_ w585] -> w564
            tunnel: w563 -> [_ w586]
            tunnel: [_ w584] -> w560
            frame False {
            }
            frame True {
              n211 = Increment(x=w586) -> (x+1=w585:dbl)
              n212 = Greater Or Equal?(x=w585, y=8.0) -> (x >= y?=w584:bool)
            }
          }
          n213 = feedback-in #8(w564) -> ()
          n214 = Greater?(x=w544, y=3) -> (0:w559:bool)
          n215 = Add(x=w570, y=w569) -> (x+y=w543:i32)
          n216 = local read "ref_t_max"() -> (w547:dbl)
          n217 = Bundle("Horizontal"=w531, "Vertical"=w540) -> (w534:cluster{"Horizontal":i32, "Vertical":i32})  [unwired: 1 in]
          n218 = Square Root(x=w543) -> (sqrt(x)=w539:dbl)
          n219 = Multiply(x=w544, y=0.01) -> (x*y=w553:dbl)
          n220 = case shown="False" w530 {
            tunnel: [w576 w580] -> w535
            tunnel: w534 -> [_ w579]
            tunnel: w533 -> [_ w578]
            tunnel: w532 -> [_ w577]
            frame False {
              n221 = call <vilib>:"Draw Circle by Radius.vi"() -> ("new picture"=w576:picture)  [unwired: 11 in]
            }
            frame True {
              n222 = local read "Cor do ponteiro"() -> (w582:u32)
              n223 = call <vilib>:"Draw Circle by Radius.vi"("color(black)"=w582, "fill?(F)"=TRUE, "pixel center"=w579, "radius"=w577, "picture"=w578) -> ("new picture"=w580:picture)  [unwired: 6 in]
            }
          }
          n224 = Insert Into Array(array=w556, new element=w539) -> (w549:dbl[])  [unwired: 1 in]
          n225 = And(x=w560, y=w559) -> (x .and. y?=w548:bool)
          n226 = Insert Into Array(array=w550, new element=w553) -> (w551:dbl[])  [unwired: 1 in]
          n227 = Insert Into Array(array=w541, new element=w540) -> (w542:i32[])  [unwired: 1 in]
          n228 = Greater?(x=w544, y=w547) -> (0:w546:bool)
          n229 = Or(x=w548, y=w546) -> (x .or. y?=w545:bool)
          n230 = Insert Into Array(array=w537, new element=w531) -> (w538:i32[])  [unwired: 1 in]
          n231 = local write "tela"(w535) -> ()
          n232 = Index Array(array=w549, index=w544) -> (element=→"ponto_final":dbl)
        }
        "Array_x" <- w513
        "Horizontal_posicao_px" <- w510
        "Vertical_posicao_px" <- w509
        n233 = call-poly <vilib>:"Close Input Device.vi"("error in (no error)"=w523, "device ID"=w522) -> ()  [unwired: 8 in, 1 out]
        n234 = Subtract(x=w516, y=8 ("x")) -> (x-y=w514:i32)
        n235 = Multiply(x=w514, y=10) -> (x*y=→"Tempo de movimento":i32)
      }
      frame #10 {
        n236 = local read "Alvo_horizontal_px"() -> (w592:dbl)
        n237 = local read "Vertical_atual_px"() -> (w590:i32)
        n238 = local read "Horizontal_atual_px"() -> (w591:i32)
        n239 = local read "Alvo_vertical_px"() -> (w589:dbl)
        n240 = local read "FB terminal"() -> (w587:bool)
        n241 = while {
          tunnel: w611 -> [w672]
          shift-right: [w663] -> _
          shift-left: 0.0 -> [w664]
          shift-right: [w662] -> w605
          shift-left: dbl[] [] -> [w661]
          i -> [w667]
          stop <- w670 stop-if-true
          n242 = Increment(x=w667) -> (x+1=w674:i32)
          n243 = Array Size(array=w672) -> (size(s)=w673:i32)
          n244 = Index Array(array=w672, index=w674) -> (element=w666:i32)
          n245 = Index Array(array=w672, index=w667) -> (element=w669:i32)
          n246 = Subtract(x=w669, y=w666) -> (x-y=w665:i32)
          n247 = Decrement(x=w673) -> (x-1=w671:i32)
          n248 = Absolute Value(x=w665) -> (abs(x)=w668:i32)
          n249 = Equal?(x=w671, y=w667) -> (x = y?=w670:bool)
          n250 = Add(x=w664, y=w668) -> (x+y=w663:dbl)
          n251 = Insert Into Array(array=w661, new element=w663) -> (w662:dbl[])  [unwired: 1 in]
        }
        n252 = case shown="True" w587 {
          frame False {
            n253 = call <vilib>:"Draw Circle by Radius.vi"() -> ("new picture"=w617:picture)  [unwired: 11 in]
            n254 = local write "tela"(w617) -> ()
          }
          frame True {
            n255 = local read "Tempo de movimento"() -> (w635:i32)
            n256 = local read "Tempo de reação"() -> (w634:i32)
            n257 = Add(x=w635, y=w634) -> (x+y=w633:i32)
            n258 = Number To Decimal String(number=w633) -> (decimal integer string=w636:string)  [unwired: 1 in]
            n259 = property on="TM" class="Str"("Visible"=TRUE) -> ()  [unwired: 2 in, 2 out]
            n260 = local write "TM"(w636) -> ()
            n261 = local read "Horizontal_posicao_px"() -> (w631:i32[])
            n262 = local read "Vertical_posicao_px"() -> (w632:i32[])
            n263 = Array Size(array=w631) -> (size(s)=w627:i32)
            n264 = Array Size(array=w632) -> (size(s)=w623:i32)
            n265 = local read "ref_pont"() -> (w620:dbl)
            n266 = Subtract(x=w627, y=1) -> (x-y=w625:i32)
            n267 = Index Array(array=w631, index=w625) -> (element=w621:i32)
            n268 = Subtract(x=w623, y=1) -> (x-y=w622:i32)
            n269 = local read "execucao"() -> (w628:picture)
            n270 = Index Array(array=w632, index=w622) -> (element=w630:i32)
            n271 = Bundle("Vertical"=w621, "Vertical"=w630) -> (w629:cluster{"Vertical":i32, "Vertical":i32})  [unwired: 1 in]
            n272 = local read "Cor do ponteiro"() -> (w618:u32)
            n273 = call <vilib>:"Draw Circle by Radius.vi"("color(black)"=w618, "fill?(F)"=TRUE, "pixel center"=w629, "radius"=w620, "picture"=w628) -> ("new picture"=w638:picture)  [unwired: 6 in]
            n274 = local write "tela"(w638) -> ()
          }
        }
        n275 = while {
          tunnel: w608 -> [w658]
          shift-right: [w649] -> _
          shift-left: 0.0 -> [w650]
          shift-right: [w648] -> w607
          shift-left: dbl[] [] -> [w647]
          i -> [w653]
          stop <- w656 stop-if-true
          n276 = Increment(x=w653) -> (x+1=w660:i32)
          n277 = Array Size(array=w658) -> (size(s)=w659:i32)
          n278 = Index Array(array=w658, index=w660) -> (element=w652:i32)
          n279 = Index Array(array=w658, index=w653) -> (element=w655:i32)
          n280 = Subtract(x=w655, y=w652) -> (x-y=w651:i32)
          n281 = Decrement(x=w659) -> (x-1=w657:i32)
          n282 = Absolute Value(x=w651) -> (abs(x)=w654:i32)
          n283 = Equal?(x=w657, y=w653) -> (x = y?=w656:bool)
          n284 = Add(x=w650, y=w654) -> (x+y=w649:dbl)
          n285 = Insert Into Array(array=w647, new element=w649) -> (w648:dbl[])  [unwired: 1 in]
        }
        n286 = Subtract(x=w589, y=w590) -> (x-y=w594:dbl)
        n287 = Subtract(x=w591, y=w592) -> (x-y=w593:dbl)
        n288 = Square(x=w594) -> (x^2=w596:dbl)
        n289 = Square(x=w593) -> (x^2=w595:dbl)
        n290 = case shown="True" TRUE {
          frame False {
          }
          frame True {
            n291 = Get Date/Time In Seconds() -> (seconds since 1Jan1904=w640:timestamp)
            n292 = Format Date/Time String(time format string (%c)="%H%M%S%4u", seconds (now)=w640) -> (date/time string=w644:string)  [unwired: 1 in]
            n293 = Fract/Exp String To Number(use system decimal point (T)=TRUE, string=w644) -> (number=w642:dbl)  [unwired: 2 in, 1 out]
            n294 = Subtract(x=w642, y=0.08) -> (x-y=→"Fim_resp":dbl)
            n295 = Seconds To Date/Time(time stamp (now)=w640) -> (date time rec=→"Fim_resp_Cluter":T1)  [unwired: 1 in]
          }
        }
        n296 = local read "Horizontal (cm/px)"() -> (w598:dbl)
        n297 = Add(x=w595, y=w596) -> (x+y=w597:dbl)
        n298 = local read "Horizontal (cm/px)"() -> (w604:dbl)
        n299 = Square Root(x=w597) -> (sqrt(x)=w599:dbl)
        n300 = local read "Horizontal (cm/px)"() -> (w606:dbl)
        n301 = Multiply(x=w599, y=w598) -> (x*y=→"erro radial (cm)":dbl)
        n302 = Multiply(x=w607, y=w606) -> (x*y=w603:dbl[])
        n303 = Multiply(x=w605, y=w604) -> (x*y=w602:dbl[])
        n304 = Square(x=w602) -> (x^2=w615:dbl[])
        n305 = Square(x=w603) -> (x^2=w614:dbl[])
        n306 = Add(x=w615, y=w614) -> (x+y=w616:dbl[])
        n307 = Square Root(x=w616) -> (sqrt(x)=w601:dbl[])
      }
      frame #11 {
        # "intervalor\nentre fim e o inicio"
        # "cortar o vetor"
        n308 = local read "Array_x"() -> (w689:dbl[])
        n309 = Array Size(array=w685) -> (size(s)=w687:i32)
        n310 = Array Size(array=w679) -> (size(s)=w683:i32)
        n311 = Array Size(array=w678) -> (size(s)=w699:i32)
        n312 = Array Size(array=w689) -> (size(s)=w694:i32)
        n313 = Subtract(x=w687, y=8) -> (x-y=w684:i32)
        n314 = Subtract(x=w683, y=8) -> (x-y=w681:i32)
        n315 = Wait (ms)(milliseconds to wait="Intervalo entre o fim e o inicio da próxima tentativa") -> ()  [unwired: 1 out]
        n316 = Subtract(x=w699, y=8) -> (x-y=w697:i32)
        n317 = Subtract(x=w694, y=8) -> (x-y=w692:i32)
        n318 = Array Subset(array=w685, index=2, length=w684) -> (w677:dbl[])
        "posicao_horizontal" <- w677
        n319 = Array Subset(array=w679, index=1, length=w681) -> (w676:dbl[])
        "posicao_vertical" <- w676
        n320 = Array Subset(array=w678, index=1, length=w697) -> (w696:dbl[])
        "posicao_total" <- w696
        n321 = Array Subset(array=w689, index=1, length=w692) -> (→"eixo x":dbl[])
      }
      frame #12 {
        n322 = Array Subset(array=w700, index=0, length=1) -> (w701:dbl[])
        n323 = Array Subset(array=w702, index=0, length=1) -> (w707:dbl[])
        n324 = Array Subset(array=w715, index=0, length=1) -> (w713:dbl[])
        n325 = Index Array(array=w701, index=0) -> (element=→"ref_p_inicial_horizontal":dbl)
        n326 = Index Array(array=w707, index=0) -> (element=→"ref_p_inicial_vertical":dbl)
        n327 = Index Array(array=w713, index=0) -> (element=→"ref_p_inicial_total":dbl)
      }
      frame #13 {
        # "Filtro"
        # "Filtro"
        n328 = local read "ref_p_inicial_total"() -> (w746:dbl)
        n329 = local read "ref_p_inicial_horizontal"() -> (w740:dbl)
        n330 = local read "ref_p_inicial_vertical"() -> (w743:dbl)
        n331 = Subtract(x=w741, y=w740) -> (x-y=w742:dbl[])
        n332 = Subtract(x=w747, y=w746) -> (x-y=w748:dbl[])
        n333 = Absolute Value(x=w742) -> (abs(x)=w730:dbl[])
        n334 = Subtract(x=w744, y=w743) -> (x-y=w745:dbl[])
        n335 = Absolute Value(x=w748) -> (abs(x)=w737:dbl[])
        n336 = Absolute Value(x=w745) -> (abs(x)=w733:dbl[])
        n337 = Array Size(array=w737) -> (size(s)=w739:i32)
        n338 = Array Size(array=w733) -> (size(s)=w735:i32)
        n339 = Array Size(array=w730) -> (size(s)=w732:i32)
        n340 = Array Subset(array=w737, index=1, length=w739) -> (→"Deslocamento_Total__bruto":dbl[])
        n341 = Array Subset(array=w733, index=1, length=w735) -> (w725:dbl[])
        "Deslocamento_Vertical_bruto" <- w725
        n342 = Array Subset(array=w730, index=1, length=w732) -> (w719:dbl[])
        "Deslocamento_Horizontal_bruto" <- w719
        n343 = call-poly <vilib>:"Butterworth Filter.vi"("order"=2, "filter type"=Filter_Passband_Type."Lowpass", "low cutoff freq: fl"=12.0, "sampling freq: fs"=100.0, "X"=w725) -> ("Filtered X"=→"Deslocamento_Vertical_fill":dbl[])  [unwired: 3 in, 1 out]
        n344 = call-poly <vilib>:"Butterworth Filter.vi"("order"=2, "filter type"=Filter_Passband_Type."Lowpass", "low cutoff freq: fl"=12.0, "sampling freq: fs"=100.0, "X"=w719) -> ("Filtered X"=→"Deslocamento_Horizontal_fill":dbl[])  [unwired: 3 in, 1 out]
      }
      frame #14 {
        # "fazendo a meta precisao"
        # "Filtro"
        n345 = local read "posicao_horizontal"() -> (w754:dbl[])
        n346 = local read "posicao_total"() -> (w753:dbl[])
        n347 = local read "Deslocamento_Total__bruto"() -> (w762:dbl[])
        n348 = local read "ref_V_alvo"() -> (w749:dbl)
        n349 = Divide(x=w754, y=w753) -> (x/y=w752:dbl[])
        n350 = local read "ref_H_alvo"() -> (w757:dbl)
        n351 = call <vilib>:"Draw Circle by Radius.vi"() -> ("new picture"=w756:picture)  [unwired: 11 in]
        n352 = Inverse Sine(1:w752) -> (0:w751:dbl[])
        n353 = call-poly <vilib>:"Butterworth Filter.vi"("order"=2, "filter type"=Filter_Passband_Type."Lowpass", "low cutoff freq: fl"=12.0, "sampling freq: fs"=100.0, "X"=w762) -> ("Filtered X"=→"Deslocamento_total_filtrado":dbl[])  [unwired: 3 in, 1 out]
        n354 = Square(x=w749) -> (x^2=w759:dbl)
        n355 = Square(x=w757) -> (x^2=w758:dbl)
        n356 = local write "tela"(w756) -> ()
        n357 = expression code="(x/pi)*180.0" "radians to degrees"(w751) -> (→"Graus":dbl[])
        n358 = Add(x=w758, y=w759) -> (x+y=w760:dbl)
        n359 = Square Root(x=w760) -> (sqrt(x)=→"meta_precisao":dbl)
      }
      frame #15 {
        n360 = local read "Deslocamento_total_filtrado"() -> (w767:dbl[])
        n361 = local read "eixo x"() -> (w768:dbl[])
        n362 = call "Convert to Dynamic Data"("Array"=w768) -> ("Dynamic Data Type"=w769:dynamicdata)  [unwired: 3 in]
        n363 = call "Convert to Dynamic Data2"("Array"=w767) -> ("Dynamic Data Type"=w770:dynamicdata)  [unwired: 3 in]
        n364 = call "deslocamento"("Y Input"=w770, "X Input"=w769) -> ("XY Graph"=→"Deslocamento":cluster{"X":dbl[], "Y":dbl[]}[])  [unwired: 8 in, 1 out]
      }
      frame #16 {
        # "Velocidade"
        # "Velocidade"
        n365 = local read "Deslocamento_total_filtrado"() -> (w788:dbl[])
        n366 = call <vilib>:"Derivative x(t).vi"("dt"=0.01, "Initial Condition"=dbl[] [0.0], "X"=w788) -> ("dX/dt"=w772:dbl[])  [unwired: 7 in, 1 out]
        n367 = local read "eixo x"() -> (w773:dbl[])
        n368 = call-poly <vilib>:"Butterworth Filter.vi"("order"=2, "filter type"=Filter_Passband_Type."Lowpass", "low cutoff freq: fl"=12.0, "sampling freq: fs"=100.0, "X"=w772) -> ("Filtered X"=w774:dbl[])  [unwired: 3 in, 1 out]
        n369 = Array Size(array=w774) -> (size(s)=w782:i32)
        n370 = call "Convert to Dynamic Data3"("Array"=w773) -> ("Dynamic Data Type"=w786:dynamicdata)  [unwired: 3 in]
        n371 = Subtract(x=w782, y=1) -> (x-y=w780:i32)
        n372 = Array Subset(array=w774, index=0, length=w780) -> (w779:dbl[])
        "Velocidade" <- w779
        n373 = call "Convert to Dynamic Data4"("Array"=w779) -> ("Dynamic Data Type"=w785:dynamicdata)  [unwired: 3 in]
        n374 = call "velocidade"("Y Input"=w785, "X Input"=w786) -> ("XY Graph"=→"Velocidade":cluster{"X":dbl[], "Y":dbl[]}[])  [unwired: 8 in, 1 out]
      }
      frame #17 {
        # "Filtro"
        # "Aceleracao"
        # "Acelracao"
        n375 = local read "Velocidade"() -> (w802:dbl[])
        n376 = call <vilib>:"Derivative x(t).vi"("dt"=0.01, "Initial Condition"=dbl[] [0.0], "X"=w802) -> ("dX/dt"=w791:dbl[])  [unwired: 7 in, 1 out]
        n377 = call-poly <vilib>:"Butterworth Filter.vi"("order"=2, "filter type"=Filter_Passband_Type."Lowpass", "low cutoff freq: fl"=12.0, "sampling freq: fs"=100.0, "X"=w791) -> ("Filtered X"=w790:dbl[])  [unwired: 3 in, 1 out]
        n378 = local read "eixo x"() -> (w803:dbl[])
        n379 = call "Convert to Dynamic Data6"("Array"=w803) -> ("Dynamic Data Type"=w807:dynamicdata)  [unwired: 3 in]
        n380 = Array Size(array=w790) -> (size(s)=w799:i32)
        n381 = Subtract(x=w799, y=2) -> (x-y=w797:i32)
        n382 = Array Subset(array=w790, index=0, length=w797) -> (w796:dbl[])
        "aceleracao" <- w796
        n383 = call "Convert to Dynamic Data5"("Array"=w796) -> ("Dynamic Data Type"=w806:dynamicdata)  [unwired: 3 in]
        n384 = call "aceleracao"("Y Input"=w806, "X Input"=w807) -> ("XY Graph"=→"Aceleracao":cluster{"X":dbl[], "Y":dbl[]}[])  [unwired: 8 in, 1 out]
      }
      frame #18 {
        # "jeark"
        n385 = local read "aceleracao"() -> (w821:dbl[])
        n386 = call <vilib>:"Derivative x(t).vi"("dt"=0.01, "Initial Condition"=dbl[] [0.0], "X"=w821) -> ("dX/dt"=w809:dbl[])  [unwired: 7 in, 1 out]
        n387 = local read "eixo x"() -> (w820:dbl[])
        n388 = call-poly <vilib>:"Butterworth Filter.vi"("order"=2, "filter type"=Filter_Passband_Type."Lowpass", "low cutoff freq: fl"=12.0, "sampling freq: fs"=100.0, "X"=w809) -> ("Filtered X"=w808:dbl[])  [unwired: 3 in, 1 out]
        n389 = Array Size(array=w808) -> (size(s)=w818:i32)
        n390 = Subtract(x=w818, y=3) -> (x-y=w816:i32)
        n391 = Array Subset(array=w808, index=0, length=w816) -> (w815:dbl[])
        "Jeark" <- w815
        n392 = call "Convert to Dynamic Data8"("Array"=w820) -> ("Dynamic Data Type"=w824:dynamicdata)  [unwired: 3 in]
        n393 = call "Convert to Dynamic Data7"("Array"=w815) -> ("Dynamic Data Type"=w810:dynamicdata)  [unwired: 3 in]
        n394 = call "jeark"("Y Input"=w810, "X Input"=w824) -> ("XY Graph"=→"Jeark":cluster{"X":dbl[], "Y":dbl[]}[])  [unwired: 8 in, 1 out]
      }
      frame #19 {
        n395 = local read "Velocidade"() -> (w828:dbl[])
        n396 = call "Convert to Dynamic Data25"("Array"=w828) -> ("Dynamic Data Type"=w827:dynamicdata)  [unwired: 3 in]
        n397 = call "Statistics"("Signals"=w827) -> ("Maximum"=→"Pico_velocidade":dynamicdata)  [unwired: 25 in, 1 out]
      }
      frame #20 {
        n398 = local read "aceleracao"() -> (w829:dbl[])
        n399 = while {
          tunnel: w829 -> [w837]
          shift-right: [w834] -> w830
          shift-left: i32[] [] -> [w833]
          i -> [w836]
          stop <- w832 stop-if-true
          w842 = 0.0 ("y")
          w846 = 0.0 ("y")
          n400 = Add(x=1, y=w836) -> (x+y=w850:i32)
          n401 = Index Array(array=w837, index=w850) -> (element=w843:dbl)
          n402 = Index Array(array=w837, index=w836) -> (element=w844:dbl)
          n403 = Less Or Equal?(x=w843, y=w846) -> (x <= y?=w848:bool)
          n404 = Greater Or Equal?(x=w843, y=w842) -> (x >= y?=w840:bool)
          n405 = Greater?(x=w844, y=w846) -> (0:w845:bool)
          n406 = Less?(x=w844, y=w842) -> (x < y?=w841:bool)
          n407 = And(x=w845, y=w848) -> (x .and. y?=w847:bool)
          n408 = And(x=w841, y=w840) -> (x .and. y?=w839:bool)
          n409 = Or(x=w847, y=w839) -> (x .or. y?=w838:bool)
          n410 = Array Size(array=w837) -> (size(s)=w835:i32)
          n411 = case shown="True" w838 {
            tunnel: w836 -> [_ w854]
            tunnel: [w851 w853] -> w834
            tunnel: w833 -> [w851 w852]
            frame False {
            }
            frame True {
              n412 = while {
                tunnel: w854 -> [w855]
                tunnel: [w858] -> w853
                tunnel: w852 -> [w859]
                i -> [w862]
                stop <- w860 stop-if-true
                n413 = Add(x=w855, y=2) -> (x+y=w856:i32)
                n414 = Equal?(x=1, y=w862) -> (x = y?=w860:bool)
                n415 = Insert Into Array(array=w859, new element=w856) -> (w858:i32[])  [unwired: 1 in]
              }
            }
          }
          n416 = Greater?(x=w836, y=w835) -> (0:w832:bool)
        }
        "ref_zero_cross" <- w830
      }
      frame #21 {
        # "posicao final em graus"
        # "Segundo ponto de correção"
        n417 = local read "Deslocamento_Vertical_fill"() -> (w864:dbl[])
        n418 = local read "ref_zero_cross"() -> (w901:i32[])
        n419 = local read "Deslocamento_total_filtrado"() -> (w879:dbl[])
        n420 = local read "Deslocamento_Horizontal_fill"() -> (w863:dbl[])
        n421 = local read "Graus"() -> (w888:dbl[])
        n422 = Array Size(array=w864) -> (size(s)=w878:i32)
        n423 = Array Size(array=w901) -> (size(s)=w900:i32)
        n424 = Array Size(array=w879) -> (size(s)=w887:i32)
        n425 = Subtract(x=w878, y=1) -> (x-y=w876:i32)
        n426 = Subtract(x=w900, y=1) -> (x-y=w898:i32)
        n427 = Array Size(array=w863) -> (size(s)=w871:i32)
        n428 = Subtract(x=w887, y=1) -> (x-y=w885:i32)
        n429 = Array Size(array=w888) -> (size(s)=w894:i32)
        n430 = Array Subset(array=w901, index=1, length=1) -> (w904:i32[])
        n431 = Array Subset(array=w864, index=w876, length=1) -> (w873:dbl[])
        n432 = Array Subset(array=w901, index=2, length=w898) -> (w897:i32[])
        n433 = Subtract(x=w871, y=1) -> (x-y=w869:i32)
        n434 = Array Subset(array=w879, index=w885, length=1) -> (w882:dbl[])
        n435 = Subtract(x=w894, y=1) -> (x-y=w892:i32)
        n436 = Index Array(array=w904, index=0) -> (element=w880:i32)
        n437 = Index Array(array=w873, index=0) -> (element=→"Posicao_final_Vertical":dbl)
        n438 = Array Subset(array=w863, index=w869, length=1) -> (w866:dbl[])
        n439 = Array Subset(array=w888, index=w892, length=1) -> (w890:dbl[])
        n440 = Multiply(x=w880, y=10) -> (x*y=→"Tempo_para_o_pico":i32)
        n441 = Index Array(array=w882, index=0) -> (element=→"Posicao_cm_final":dbl)
        n442 = Array Size(array=w897) -> (size(s)=→"n_correcoes":i32)
        n443 = Index Array(array=w890, index=0) -> (element=→"Posicao_graus_final":dbl)
        n444 = Index Array(array=w866, index=0) -> (element=→"Posicao_final_horizontal":dbl)
      }
      frame #22 {
        n445 = local read "Deslocamento_total_filtrado"() -> (w918:dbl[])
        n446 = local read "Deslocamento_Vertical_fill"() -> (w934:dbl[])
        n447 = local read "Tempo_para_o_pico"() -> (w943:i32)
        n448 = local read "Horizontal (cm/px)"() -> (w946:dbl)
        n449 = local read "Deslocamento_Horizontal_fill"() -> (w929:dbl[])
        n450 = local read "Tempo_para_o_pico"() -> (w947:i32)
        n451 = local read "meta_precisao"() -> (w945:dbl)
        n452 = local read "Graus"() -> (w949:dbl[])
        n453 = local read "Tempo de movimento"() -> (w964:i32)
        n454 = Array Subset(array=w918, index=w916, length=1) -> (w938:dbl[])
        n455 = local read "aceleracao"() -> (w923:dbl[])
        n456 = local read "Inicio_da_resposta"() -> (w941:dbl)
        n457 = local read "aceleracao"() -> (w915:dbl[])
        n458 = Index Array(array=w938, index=0) -> (element=w957:dbl)
        n459 = Array Size(array=w918) -> (size(s)=w919:i32)
        n460 = Array Subset(array=w949, index=w928, length=1) -> (w951:dbl[])
        n461 = Array Size(array=w923) -> (size(s)=w922:i32)
        n462 = Array Subset(array=w918, index=w928, length=1) -> (w955:dbl[])
        n463 = Multiply(x=w945, y=w946) -> (x*y=w944:dbl)
        n464 = Multiply(x=w947, y=100) -> (x*y=w963:i32)
        n465 = Divide(x=w943, y=1000) -> (x/y=w940:dbl)
        n466 = Subtract(x=w957, y=w944) -> (x-y=w959:dbl)
        n467 = Index Array(array=w951, index=0) -> (element=→"Posicao_graus_2_sub":dbl)
        n468 = Array Subset(array=w923, index=w916, length=w922) -> (w921:dbl[])
        n469 = Index Array(array=w955, index=0) -> (element=→"Posicao_cm_2_sub":dbl)
        n470 = Absolute Value(x=w959) -> (abs(x)=→"ER_no_2_sub":dbl)
        n471 = Divide(x=w963, y=w964) -> (x/y=→"Tempo_relativo_pico":dbl)
        n472 = Array Subset(array=w929, index=w928, length=1) -> (w926:dbl[])
        n473 = Array Subset(array=w915, index=0, length=w916) -> (w913:dbl[])
        n474 = Array Subset(array=w918, index=w916, length=w919) -> (→"Deslocamento_tototal_2_sub":dbl[])
        n475 = Array Subset(array=w934, index=w928, length=1) -> (w931:dbl[])
        n476 = Add(x=w941, y=w940) -> (x+y=→"2_sub_mov":dbl)
        n477 = Array Subset(array=w918, index=0, length=w916) -> (→"Deslocamento_tototal_1_sub":dbl[])
        n478 = call-poly <vilib>:"Numeric Integration.vi"("dt"=0.01, "Input Array"=w921) -> ("result"=w910:dbl)  [unwired: 1 in, 1 out]
        n479 = Index Array(array=w926, index=0) -> (element=→"Posicao_Hori_2_sub":dbl)
        n480 = Absolute Value(x=w910) -> (abs(x)=→"Area_acel_2_sub":dbl)
        n481 = Index Array(array=w931, index=0) -> (element=→"Posicao_vert_2_sub":dbl)
        n482 = call-poly <vilib>:"Numeric Integration.vi"("dt"=0.01, "Input Array"=w913) -> ("result"=w912:dbl)  [unwired: 1 in, 1 out]
        n483 = Absolute Value(x=w912) -> (abs(x)=→"Area_acel_1_sub":dbl)
      }
      frame #23 {
        w1074 = ".txt" ("string")
        n484 = local read "Deslocamento_tototal_2_sub"() -> (w979:dbl[])
        n485 = local read "Fim_do_warning_Cluter"() -> (w1016:T1)
        n486 = local read "Inicio_da_resposta_Cluter"() -> (w998:T1)
        n487 = local read "Deslocamento_tototal_1_sub"() -> (w981:dbl[])
        n488 = local read "posicao_total"() -> (w1050:dbl[])
        n489 = local read "Deslocamento_Horizontal_bruto"() -> (w1047:dbl[])
        n490 = local read "posicao_vertical"() -> (w1049:dbl[])
        n491 = local read "Velocidade"() -> (w1052:dbl[])
        n492 = local read "Deslocamento_Vertical_bruto"() -> (w1048:dbl[])
        n493 = local read "Inicio_do_warning_Cluter"() -> (w1025:T1)
        n494 = local read "Deslocamento_total_filtrado"() -> (w1070:dbl[])
        n495 = local read "aceleracao"() -> (w1051:dbl[])
        n496 = local read "Deslocamento_Total__bruto"() -> (w1060:dbl[])
        n497 = local read "Digite aqui o endereço e nome do arquivo"() -> (w969:string)
        n498 = local read "posicao_horizontal"() -> (w1062:dbl[])
        n499 = local read "Jeark"() -> (w1066:dbl[])
        n500 = local read "Tempo_para_o_pico"() -> (w984:i32)
        n501 = local read "tentativa"() -> (w1071:i32)
        n502 = local read "Vertical_posicao_px"() -> (w1056:i32[])
        n503 = local read "Horizontal_posicao_px"() -> (w1054:i32[])
        n504 = local read "Graus"() -> (w1044:dbl[])
        n505 = local read "Apresentacao_do_estimulo_Cluter"() -> (w1007:T1)
        n506 = Unbundle(w998) -> ("fractional second"=w1004:dbl, "second"=w1003:i32, "minute"=w1006:i32, "hour"=w1000:i32)  [unwired: 6 out]
        n507 = Concatenate Strings(w969, "_tentativa_" ("string")) -> (w1045:string)
        n508 = Unbundle(w1016) -> ("fractional second"=w1022:dbl, "second"=w1021:i32, "minute"=w1024:i32, "hour"=w1018:i32)  [unwired: 6 out]
        n509 = Format Into String(w1071) -> (resulting string=w1075:string)  [unwired: 3 in, 1 out]
        n510 = Multiply(x=w1006, y=60) -> (x*y=w1002:i32)
        n511 = Divide(x=w984, y=1000) -> (x/y=w982:dbl)
        n512 = Multiply(x=w1000, y=3600) -> (x*y=w1001:i32)
        n513 = Unbundle(w1025) -> ("fractional second"=w1031:dbl, "second"=w1030:i32, "minute"=w1033:i32, "hour"=w1027:i32)  [unwired: 6 out]
        n514 = local read "INICIO_Cluter"() -> (w1036:T1)
        n515 = Concatenate Strings(w1045, w1075) -> (w966:string)
        n516 = Multiply(x=w1024, y=60) -> (x*y=w1020:i32)
        n517 = Multiply(x=w1018, y=3600) -> (x*y=w1019:i32)
        n518 = Compound Arithmetic op=ADD(w1004, w1003, w1002, w1001) -> (w983:dbl)
        "Inicio_da_reposta(s)" <- w983
        n519 = call "Convert to Dynamic Data9"("Array"=w1070) -> ("Dynamic Data Type"=w1069:dynamicdata)  [unwired: 3 in]
        n520 = call "Convert to Dynamic Data15"("Array"=w1051) -> ("Dynamic Data Type"=w1067:dynamicdata)  [unwired: 3 in]
        n521 = call "Convert to Dynamic Data16"("Array"=w1066) -> ("Dynamic Data Type"=w1065:dynamicdata)  [unwired: 3 in]
        n522 = call "Convert to Dynamic Data14"("Array"=w1052) -> ("Dynamic Data Type"=w1068:dynamicdata)  [unwired: 3 in]
        n523 = call "Convert to Dynamic Data18"("Array"=w1049) -> ("Dynamic Data Type"=w1063:dynamicdata)  [unwired: 3 in]
        n524 = call "Convert to Dynamic Data19"("Array"=w1062) -> ("Dynamic Data Type"=w1061:dynamicdata)  [unwired: 3 in]
        n525 = Multiply(x=w1033, y=60) -> (x*y=w1029:i32)
        n526 = local read "Fim_resp_Cluter"() -> (w990:T1)
        n527 = call "Convert to Dynamic Data17"("Array"=w1050) -> ("Dynamic Data Type"=w1064:dynamicdata)  [unwired: 3 in]
        n528 = call "Convert to Dynamic Data20"("Array"=w1060) -> ("Dynamic Data Type"=w1059:dynamicdata)  [unwired: 3 in]
        n529 = Multiply(x=w1027, y=3600) -> (x*y=w1028:i32)
        n530 = Concatenate Strings(w966, w1074) -> (w1073:string)
        n531 = Compound Arithmetic op=ADD(w1022, w1021, w1020, w1019) -> (→"Fim_do_warning(s)":dbl)
        n532 = call "Convert to Dynamic Data21"("Array"=w1048) -> ("Dynamic Data Type"=w1058:dynamicdata)  [unwired: 3 in]
        n533 = Add(x=w983, y=w982) -> (x+y=→"2_sub_mov(s)":dbl)
        n534 = Concatenate Strings(w969, w1074) -> (w1072:string)
        n535 = call "Convert to Dynamic Data22"("Array"=w1047) -> ("Dynamic Data Type"=w1057:dynamicdata)  [unwired: 3 in]
        n536 = call "Convert to Dynamic Data23"("Array"=w1056) -> ("Dynamic Data Type"=w1055:dynamicdata)  [unwired: 3 in]
        n537 = call "Convert to Dynamic Data24"("Array"=w1054) -> ("Dynamic Data Type"=w1053:dynamicdata)  [unwired: 3 in]
        n538 = Compound Arithmetic op=ADD(w1031, w1030, w1029, w1028) -> (→"Inicio_do_warning(s)":dbl)
        n539 = String To Path(string=w1072) -> (path=→"referencia de endereco":path)
        n540 = call "Convert to Dynamic Data29"("Array"=w1044) -> ("Dynamic Data Type"=w1043:dynamicdata)  [unwired: 3 in]
        n541 = Unbundle(w1036) -> ("fractional second"=w1040:dbl, "second"=w1039:i32, "minute"=w1042:i32, "hour"=w1035:i32)  [unwired: 6 out]
        n542 = String To Path(string=w1073) -> (path=w1076:path)
        n543 = Unbundle(w1007) -> ("fractional second"=w1013:dbl, "second"=w1012:i32, "minute"=w1015:i32, "hour"=w1009:i32)  [unwired: 6 out]
        n544 = Unbundle(w990) -> ("fractional second"=w995:dbl, "second"=w977:i32, "minute"=w997:i32, "hour"=w992:i32)  [unwired: 6 out]
        n545 = call "Convert to Dynamic Data51"("Array"=w979) -> ("Dynamic Data Type"=w978:dynamicdata)  [unwired: 3 in]
        n546 = call "Convert to Dynamic Data50"("Array"=w981) -> ("Dynamic Data Type"=w980:dynamicdata)  [unwired: 3 in]
        n547 = Concatenate Strings(w966, ".xls" ("string")) -> (w972:string)
        n548 = Multiply(x=w1042, y=60) -> (x*y=w1038:i32)
        n549 = Multiply(x=w1015, y=60) -> (x*y=w1011:i32)
        n550 = Multiply(x=w1035, y=3600) -> (x*y=w1037:i32)
        n551 = Multiply(x=w1009, y=3600) -> (x*y=w1010:i32)
        n552 = Merge Signals(w1069, w1068, w1067, w1065, w1064, w1063, w1061, w1059, w1058, w1057, w1055, w1053, w1043, w980, w978) -> (w970:dynamicdata)
        n553 = Multiply(x=w997, y=60) -> (x*y=w994:i32)
        n554 = Multiply(x=w992, y=3600) -> (x*y=w993:i32)
        n555 = String To Path(string=w972) -> (path=w971:path)
        n556 = Compound Arithmetic op=ADD(w1040, w1039, w1038, w1037) -> (→"INICIO(s)":dbl)
        n557 = Compound Arithmetic op=ADD(w1013, w1012, w1011, w1010) -> (→"Apresentacao_do_estimulo(s)":dbl)
        n558 = Compound Arithmetic op=ADD(w995, w977, w994, w993) -> (w974:dbl)
        n559 = call "Salvar em xls"("Signals"=w970, "Filename"=w971) -> ()  [unwired: 15 in, 3 out]
        n560 = call "Salvar em txt"("Signals"=w970, "Filename"=w1076) -> ()  [unwired: 15 in, 3 out]
        n561 = Subtract(x=w974, y=0.08) -> (x-y=→"Fim_da_reposta(s)":dbl)
      }
      frame #24 {
        n562 = local read "Horizontal (cm/px)"() -> (w1090:dbl)
        n563 = local read "Horizontal"() -> (w1086:dbl)
        n564 = local read "ref_V_alvo"() -> (w1091:dbl)
        n565 = local read "ref_H_alvo"() -> (w1092:dbl)
        n566 = local read "Apresentacao_do_estimulo"() -> (w1109:dbl)
        n567 = local read "Apresentacao_do_estimulo(s)"() -> (w1102:dbl)
        n568 = local read "Inicio_da_reposta(s)"() -> (w1101:dbl)
        n569 = local read "Area_acel_2_sub"() -> (w1094:dbl)
        n570 = local read "Posicao_final_horizontal"() -> (w1098:dbl)
        n571 = local read "Inicio_do_warning(s)"() -> (w1104:dbl)
        n572 = local read "Inicio_da_resposta"() -> (w1108:dbl)
        n573 = local read "Fim_do_warning(s)"() -> (w1103:dbl)
        n574 = local read "Vertical  (cm)"() -> (w1089:dbl)
        n575 = local read "Fim_do_warning"() -> (w1110:dbl)
        n576 = local read "Posicao_final_Vertical"() -> (w1097:dbl)
        n577 = local read "Horizontal_atual_px"() -> (w1080:i32)
        n578 = local read "Fim_da_reposta(s)"() -> (w1099:dbl)
        n579 = local read "Alvo_horizontal_px"() -> (w1078:dbl)
        n580 = local read "Inicio_do_warning"() -> (w1111:dbl)
        n581 = local read "Tempo de movimento"() -> (w1124:i32)
        n582 = local read "Vertical_atual_px"() -> (w1079:i32)
        n583 = local read "Tempo de reação"() -> (w1125:i32)
        n584 = local read "INICIO"() -> (w1112:dbl)
        n585 = local read "2_sub_mov(s)"() -> (w1100:dbl)
        n586 = local read "Posicao_Hori_2_sub"() -> (w1096:dbl)
        n587 = local read "2_sub_mov"() -> (w1107:dbl)
        n588 = local read "Alvo_vertical_px"() -> (w1077:dbl)
        n589 = local read "INICIO(s)"() -> (w1105:dbl)
        n590 = local read "Tempo_relativo_pico"() -> (w1121:dbl)
        n591 = local read "Posicao_graus_2_sub"() -> (w1114:dbl)
        n592 = local read "Posicao_cm_final"() -> (w1117:dbl)
        n593 = local read "Tempo_para_o_pico"() -> (w1113:i32)
        n594 = local read "Posicao_vert_2_sub"() -> (w1095:dbl)
        n595 = local read "Posicao_cm_2_sub"() -> (w1115:dbl)
        n596 = local read "Pico_velocidade"() -> (w1120:dbl)
        n597 = local read "Posicao_graus_final"() -> (w1118:dbl)
        n598 = local read "erro radial (cm)"() -> (w1122:dbl)
        n599 = local read "ER_no_2_sub"() -> (w1116:dbl)
        n600 = local read "Area_acel_1_sub"() -> (w1093:dbl)
        n601 = local read "n_correcoes"() -> (w1119:i32)
        n602 = local read "Fim_resp"() -> (w1106:dbl)
        n603 = Multiply(x=w1092, y=w1090) -> (x*y=w1087:dbl)
        n604 = local read "Vertical"() -> (w1084:dbl)
        n605 = local read "codigo"() -> (w1081:dbl)
        n606 = Multiply(x=w1091, y=w1090) -> (x*y=w1088:dbl)
        n607 = Subtract(x=w1087, y=w1086) -> (x-y=w1085:dbl)
        n608 = Add(x=w1125, y=w1124) -> (x+y=w1123:i32)
        n609 = Subtract(x=w1089, y=w1088) -> (x-y=w1083:dbl)
        n610 = Subtract(x=w1083, y=w1084) -> (x-y=w1082:dbl)
      }
    }
  }
  n611 = call "Convert to Dynamic Data27"("Array"=w71) -> ("Dynamic Data Type"=w70:dynamicdata)  [unwired: 3 in]
  n612 = call "Convert to Dynamic Data13"("Array"=w75) -> ("Dynamic Data Type"=w74:dynamicdata)  [unwired: 3 in]
  n613 = call "Convert to Dynamic Data10"("Array"=w81) -> ("Dynamic Data Type"=w80:dynamicdata)  [unwired: 3 in]
  n614 = call "Convert to Dynamic Data12"("Array"=w77) -> ("Dynamic Data Type"=w76:dynamicdata)  [unwired: 3 in]
  n615 = call "Convert to Dynamic Data26"("Array"=w73) -> ("Dynamic Data Type"=w72:dynamicdata)  [unwired: 3 in]
  n616 = call "Convert to Dynamic Data30"("Array"=w67) -> ("Dynamic Data Type"=w66:dynamicdata)  [unwired: 3 in]
  n617 = call "Convert to Dynamic Data28"("Array"=w69) -> ("Dynamic Data Type"=w68:dynamicdata)  [unwired: 3 in]
  n618 = call "Convert to Dynamic Data11"("Array"=w79) -> ("Dynamic Data Type"=w78:dynamicdata)  [unwired: 3 in]
  n619 = call "Convert to Dynamic Data31"("Array"=w65) -> ("Dynamic Data Type"=w64:dynamicdata)  [unwired: 3 in]
  n620 = call "Convert to Dynamic Data33"("Array"=w61) -> ("Dynamic Data Type"=w60:dynamicdata)  [unwired: 3 in]
  n621 = call "Convert to Dynamic Data32"("Array"=w63) -> ("Dynamic Data Type"=w62:dynamicdata)  [unwired: 3 in]
  n622 = call "Convert to Dynamic Data34"("Array"=w59) -> ("Dynamic Data Type"=w58:dynamicdata)  [unwired: 3 in]
  n623 = call "Convert to Dynamic Data35"("Array"=w57) -> ("Dynamic Data Type"=w56:dynamicdata)  [unwired: 3 in]
  n624 = call "Convert to Dynamic Data37"("Array"=w52) -> ("Dynamic Data Type"=w53:dynamicdata)  [unwired: 3 in]
  n625 = call "Convert to Dynamic Data36"("Array"=w55) -> ("Dynamic Data Type"=w54:dynamicdata)  [unwired: 3 in]
  n626 = call "Convert to Dynamic Data38"("Array"=w51) -> ("Dynamic Data Type"=w50:dynamicdata)  [unwired: 3 in]
  n627 = call "Convert to Dynamic Data39"("Array"=w48) -> ("Dynamic Data Type"=w49:dynamicdata)  [unwired: 3 in]
  n628 = call "Convert to Dynamic Data40"("Array"=w47) -> ("Dynamic Data Type"=w46:dynamicdata)  [unwired: 3 in]
  n629 = call "Convert to Dynamic Data41"("Array"=w45) -> ("Dynamic Data Type"=w44:dynamicdata)  [unwired: 3 in]
  n630 = call "Convert to Dynamic Data42"("Array"=w43) -> ("Dynamic Data Type"=w42:dynamicdata)  [unwired: 3 in]
  n631 = call "Convert to Dynamic Data43"("Array"=w41) -> ("Dynamic Data Type"=w40:dynamicdata)  [unwired: 3 in]
  n632 = call "Convert to Dynamic Data44"("Array"=w39) -> ("Dynamic Data Type"=w38:dynamicdata)  [unwired: 3 in]
  n633 = call "Convert to Dynamic Data45"("Array"=w37) -> ("Dynamic Data Type"=w36:dynamicdata)  [unwired: 3 in]
  n634 = call "Convert to Dynamic Data47"("Array"=w32) -> ("Dynamic Data Type"=w33:dynamicdata)  [unwired: 3 in]
  n635 = call "Convert to Dynamic Data46"("Array"=w35) -> ("Dynamic Data Type"=w34:dynamicdata)  [unwired: 3 in]
  n636 = call "Convert to Dynamic Data48"("Array"=w30) -> ("Dynamic Data Type"=w31:dynamicdata)  [unwired: 3 in]
  n637 = call "Convert to Dynamic Data49"("Array"=w29) -> ("Dynamic Data Type"=w28:dynamicdata)  [unwired: 3 in]
  n638 = call "Convert to Dynamic Data52"("Array"=w27) -> ("Dynamic Data Type"=w21:dynamicdata)  [unwired: 3 in]
  n639 = call "Convert to Dynamic Data53"("Array"=w26) -> ("Dynamic Data Type"=w25:dynamicdata)  [unwired: 3 in]
  n640 = call "Convert to Dynamic Data54"("Array"=w24) -> ("Dynamic Data Type"=w23:dynamicdata)  [unwired: 3 in]
  n641 = call "Convert to Dynamic Data55"("Array"=w22) -> ("Dynamic Data Type"=w20:dynamicdata)  [unwired: 3 in]
  n642 = call "Convert to Dynamic Data56"("Array"=w13) -> ("Dynamic Data Type"=w14:dynamicdata)  [unwired: 3 in]
  n643 = call "Convert to Dynamic Data57"("Array"=w19) -> ("Dynamic Data Type"=w18:dynamicdata)  [unwired: 3 in]
  n644 = call "Convert to Dynamic Data58"("Array"=w17) -> ("Dynamic Data Type"=w12:dynamicdata)  [unwired: 3 in]
  n645 = call "Convert to Dynamic Data59"("Array"=w16) -> ("Dynamic Data Type"=w15:dynamicdata)  [unwired: 3 in]
  n646 = call "Convert to Dynamic Data60"("Array"=w9) -> ("Dynamic Data Type"=w11:dynamicdata)  [unwired: 3 in]
  n647 = call "Convert to Dynamic Data61"("Array"=w8) -> ("Dynamic Data Type"=w7:dynamicdata)  [unwired: 3 in]
  n648 = call "Convert to Dynamic Data62"("Array"=w6) -> ("Dynamic Data Type"=w5:dynamicdata)  [unwired: 3 in]
  n649 = call "Convert to Dynamic Data63"("Array"=w4) -> ("Dynamic Data Type"=w3:dynamicdata)  [unwired: 3 in]
  n650 = call "Convert to Dynamic Data64"("Array"=w2) -> ("Dynamic Data Type"=w1:dynamicdata)  [unwired: 3 in]
  n651 = Merge Signals(w80, w78, w76, w74, w72, w70, w68, w66, w64, w62, w60, w58, w56, w54, w53, w50, w49, w46, w44, w42, w40, w38, w36, w34, w33, w31, w28, w21, w25, w23, w20, w14, w18, w12, w15, w11, w7, w5, w3, w1) -> (w82:dynamicdata)
  n652 = call "Dados Brutos"("Signals"=w82) -> ("Table"=w84:string[][])  [unwired: 4 in, 6 out]
  n653 = Fract/Exp String To Number(string=w84) -> (number=w85:dbl[][])  [unwired: 3 in, 1 out]
  n654 = call-poly <vilib>:"Write Delimited Spreadsheet.vi"("format (%.3f)"="%.3f", "2D data"=w85) -> ()  [unwired: 12 in, 2 out]
